vi "report.vi"() -> ()   [LabVIEW 2019, in "database.lvlib"]
uses:
  database.lvlib
  <vilib>/Utility/NIReport.llb/Report Type.ctl
  <vilib>/addons/_office/_exclsub.llb/font.ctl
  <vilib>/Utility/miscctls.llb/LVRowAndColumnTypeDef.ctl
  <vilib>/addons/_office/excel.llb/Excel Easy Table (str).vi
  <vilib>/Utility/NIReport.llb/NI_report.lvclass
  <vilib>/addons/_office/NI_ReportGenerationToolkit.lvlib
  <vilib>/Utility/NIReport.llb/NI_ReportGenerationCore.lvlib
panel:
  in  "Tab Control 1":T1(tab)
  in  "Tab Control 2":T2(tab)
  out "Grading Table Disc 1":string[][](table)
  out "Grading Table Disc 2":string[][](table)
  out "Grading Table Disc 3":string[][](table)
  out "Grading Table Disc 4":string[][](table)
  out "Grading Table Disc 5":string[][](table)
  out "Grading Table Disc 6":string[][](table)
  in  "Search 1":bool
  in  "Print 1":bool
  in  "Close 1":bool
  in  "Save 1":bool
  in  "Tab Control 3":T2(tab)
  out "Main Grading Table Disc 1":string[][](table)
  out "Main Grading Table Disc 2":string[][](table)
  out "Main Grading Table Disc 3":string[][](table)
  out "Main Grading Table Disc 4":string[][](table)
  out "Main Grading Table Disc 5":string[][](table)
  out "Main Grading Table Disc 6":string[][](table)
  in  "Close 2":bool
  in  "Print 2":bool
  in  "Search 2":bool
  in  "Save 2":bool
  out "Log Table":string[][](table)
  out "Log Catalog Table":string[][](table)
  in  "Search 3":bool
  in  "Print 3":bool
  in  "Close 3":bool
  in  "Save 3":bool
  out "User Table":string[][](table)
  in  "Close 4":bool
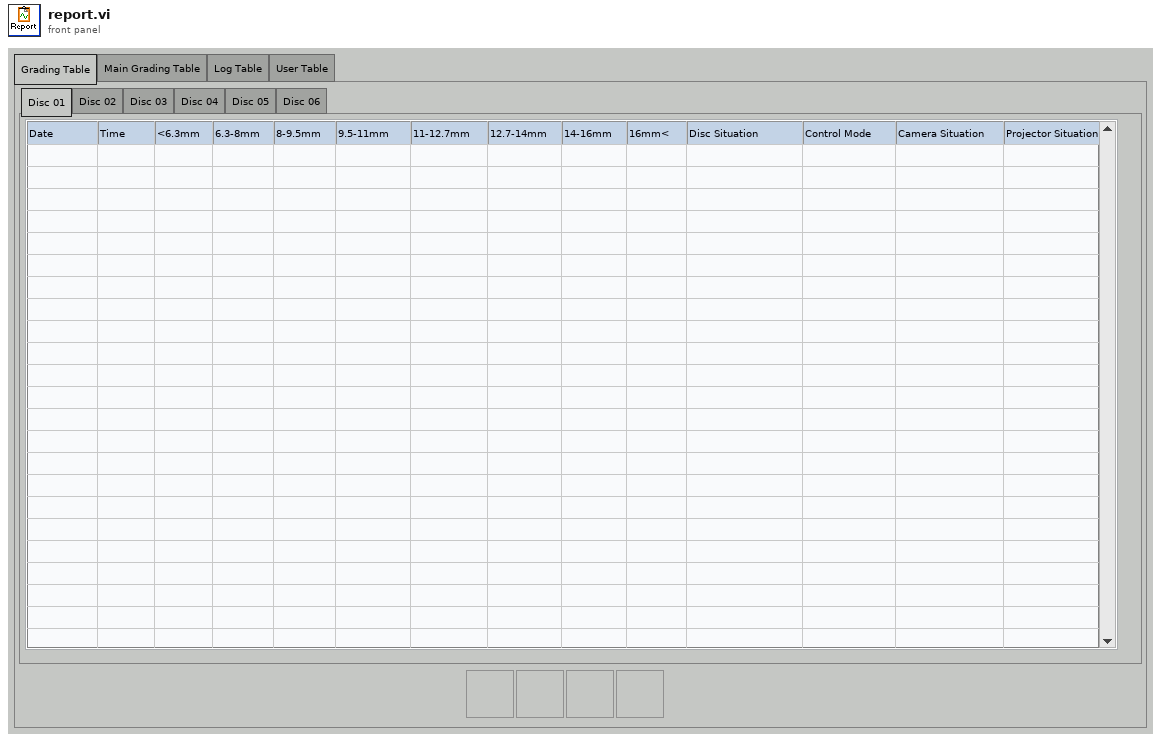
[diagram p1: front panel]
types:
  T1 = enum32{"Grading Table", "Main Grading Table", "Log Table", "User Table"}
  T2 = enum32{"Disc 01", "Disc 02", "Disc 03", "Disc 04", "Disc 05", "Disc 06"}
  T3 = enum16{"None", "On Hover", "On Key Focus", "On Hover or Key Focus"}
  T4 = typedef "NI_ReportGenerationToolkit.lvlib/font.ctl" = cluster{"font name":string, "font size":dbl, "bold":u16, "italic":u16, "underline":u16, "strike through":u16, "font color":u32}
  T5 = typedef "NI_ReportGenerationCore.lvlib/Report Type.ctl" = enum16{"HTML", "Word", "Excel"}
  T6 = enum16{"maximized", "minimized", "normal", "no change"}
  T7 = typedef "LVRowAndColumnTypeDef.ctl" = cluster{"Row":i32, "Column":i32}
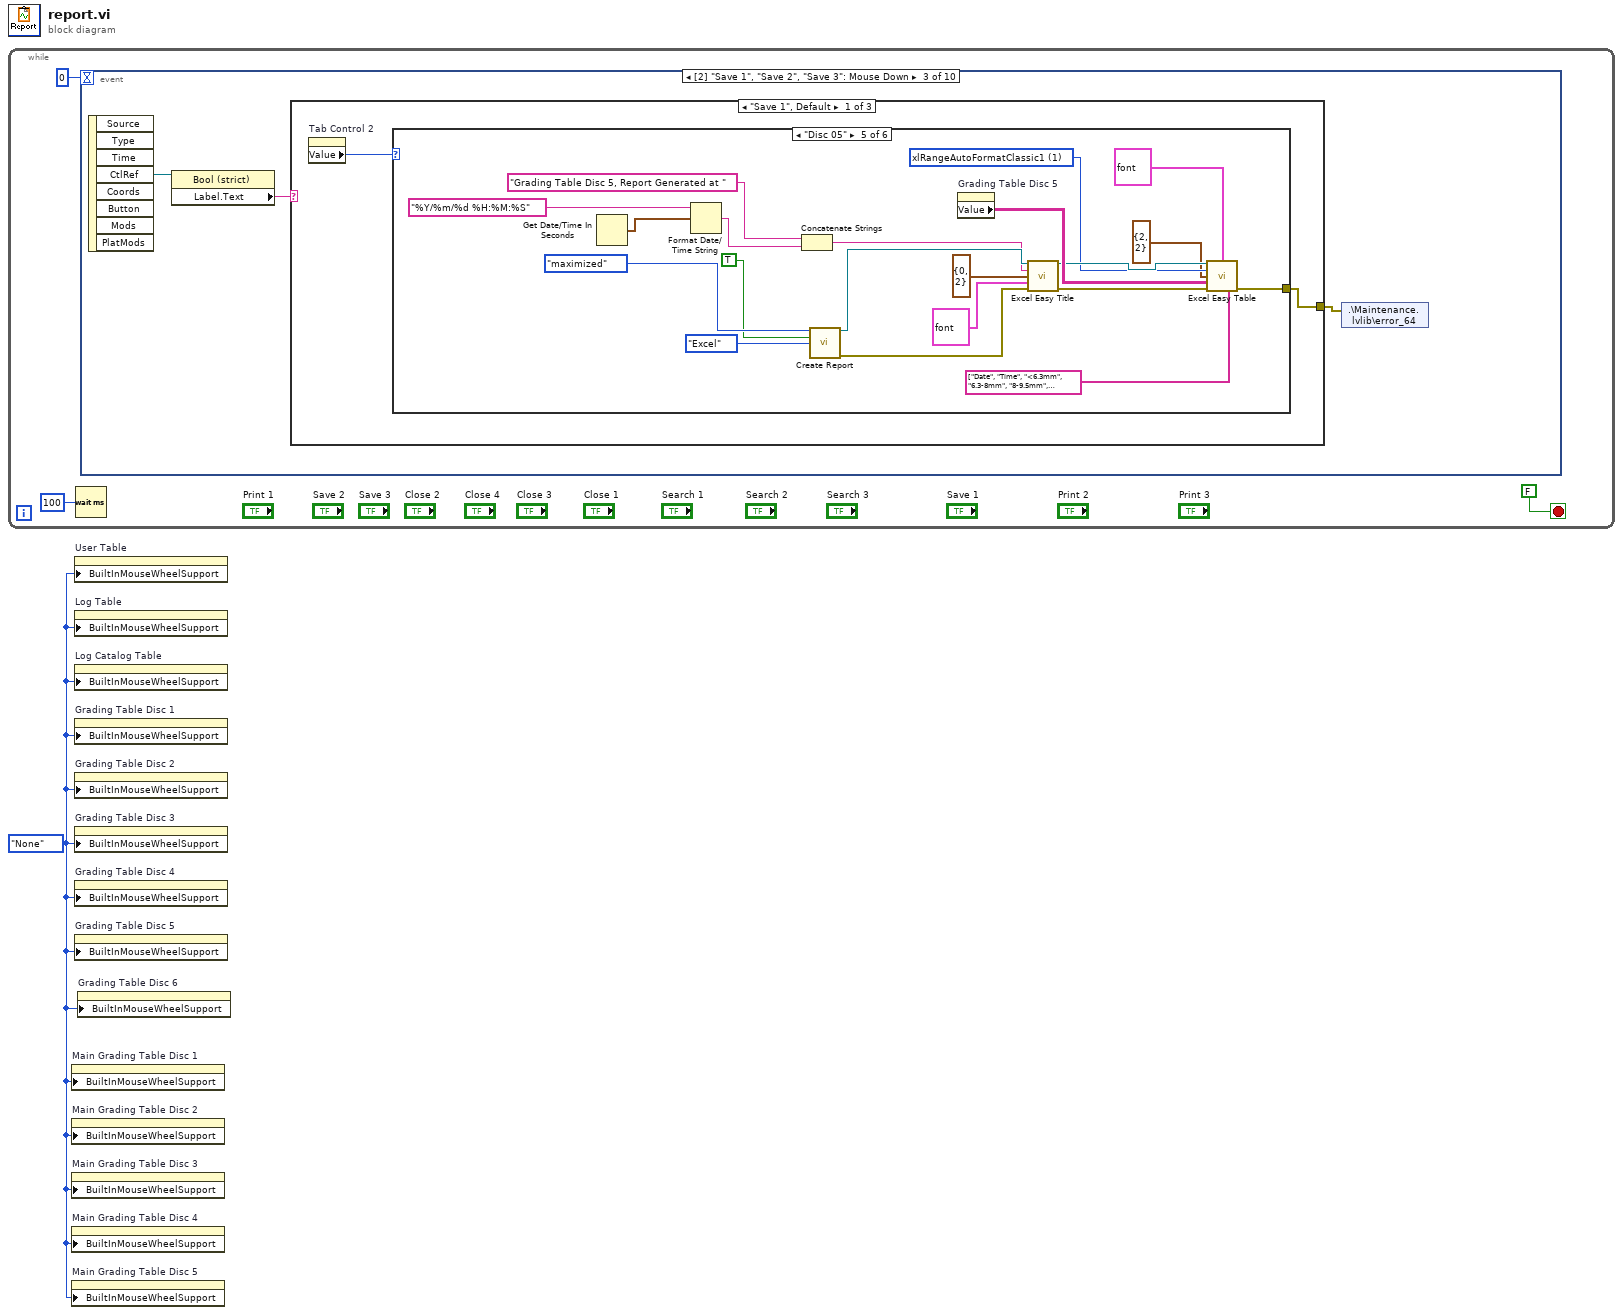
[diagram p0: block diagram]
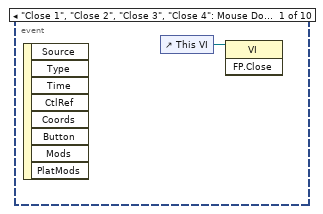
[diagram p2: hidden frame]
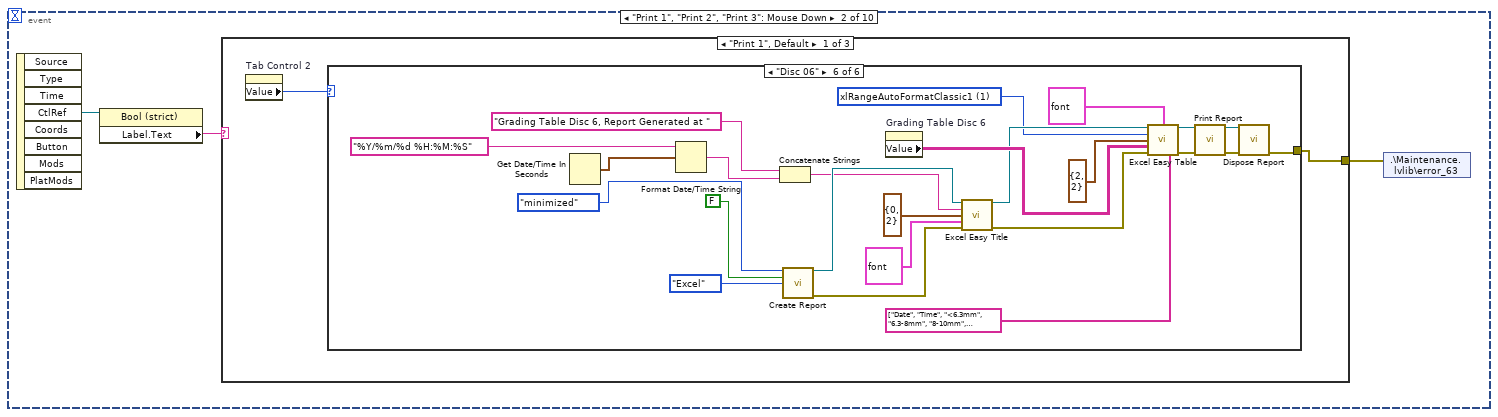
[diagram p3: hidden frame]
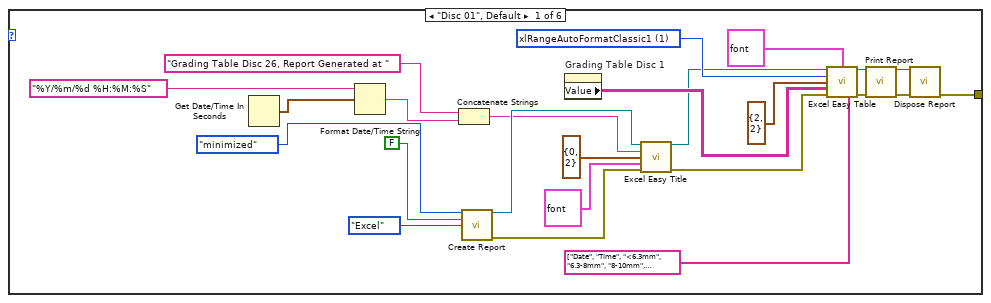
[diagram p4: hidden frame]
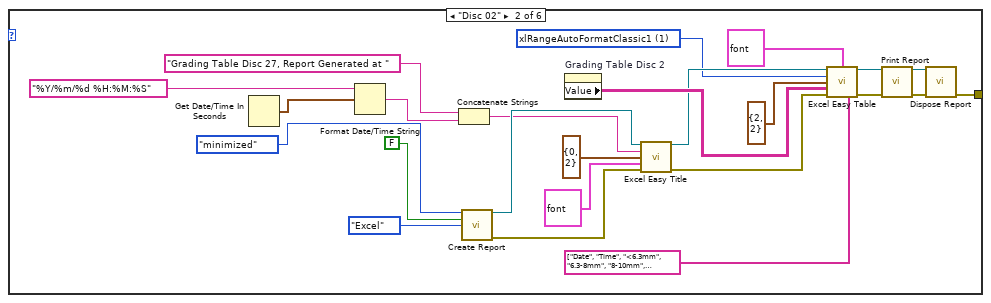
[diagram p5: hidden frame]
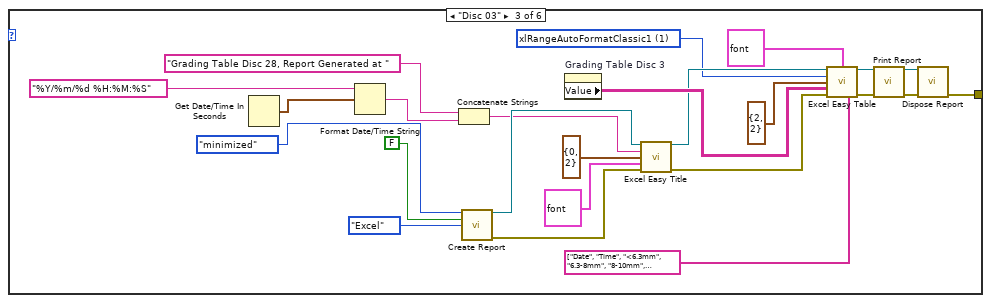
[diagram p6: hidden frame]
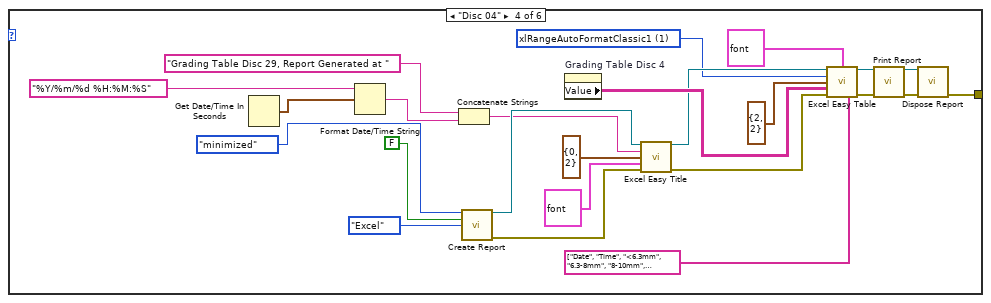
[diagram p7: hidden frame]
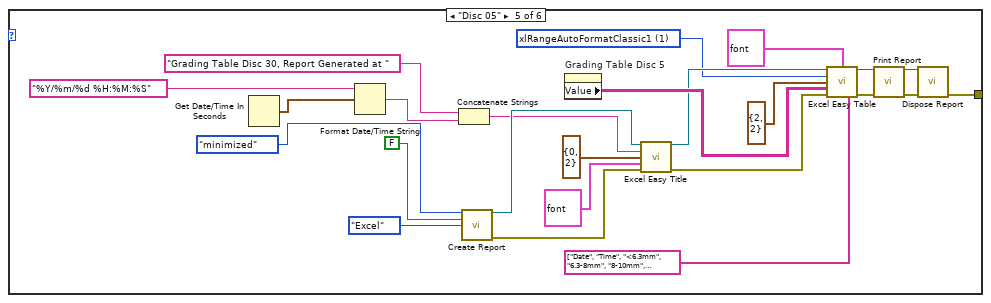
[diagram p8: hidden frame]
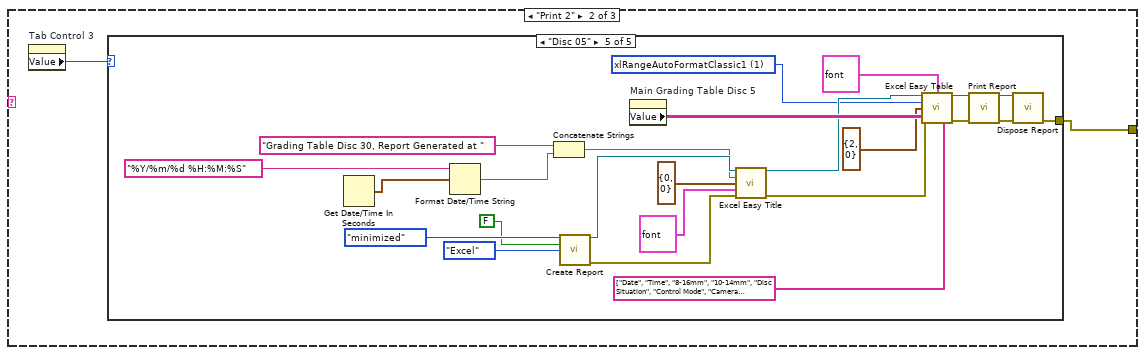
[diagram p9: hidden frame]
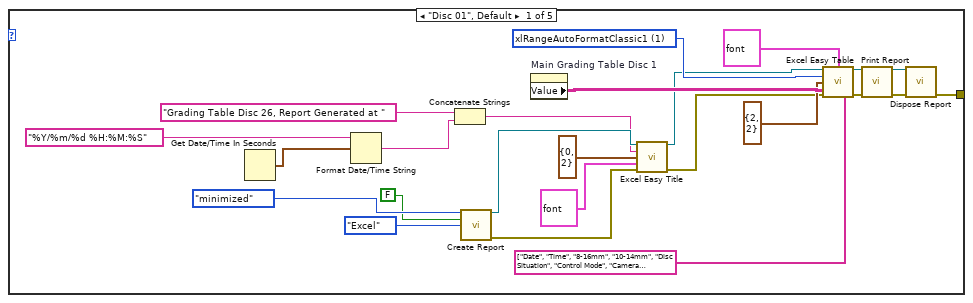
[diagram p10: hidden frame]
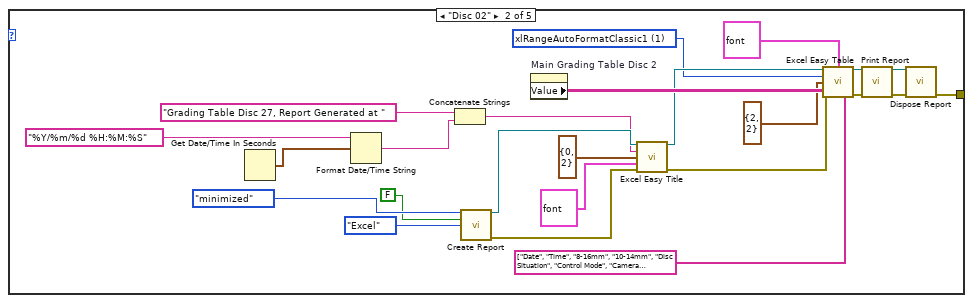
[diagram p11: hidden frame]
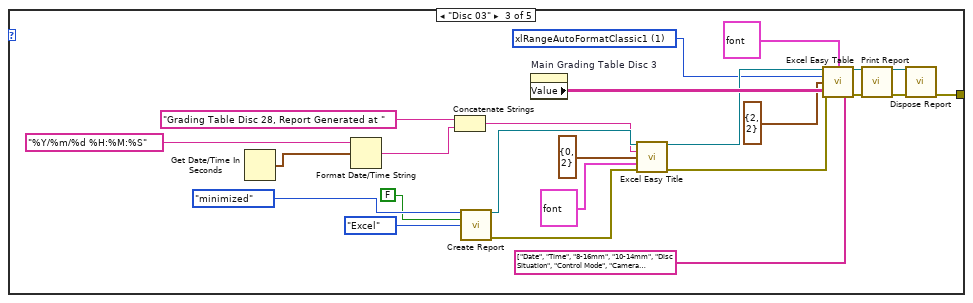
[diagram p12: hidden frame]
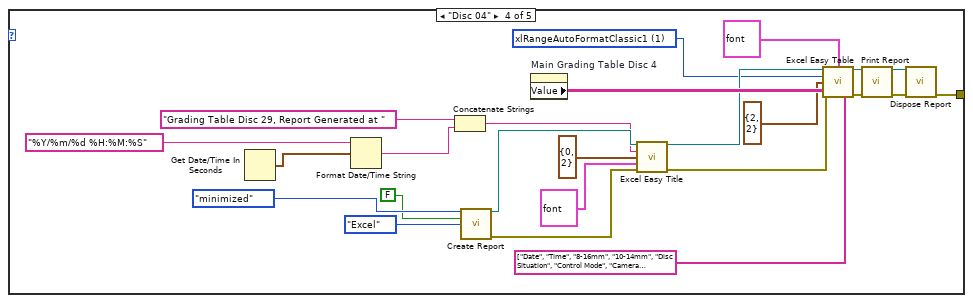
[diagram p13: hidden frame]
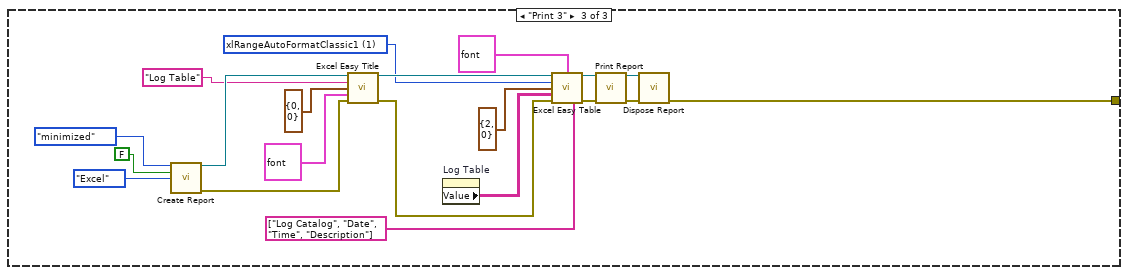
[diagram p14: hidden frame]
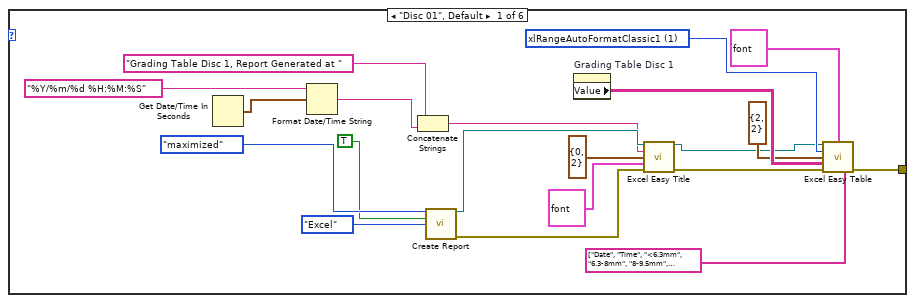
[diagram p15: hidden frame]
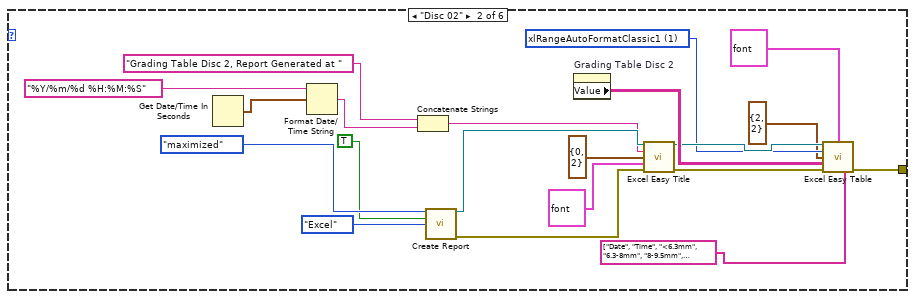
[diagram p16: hidden frame]
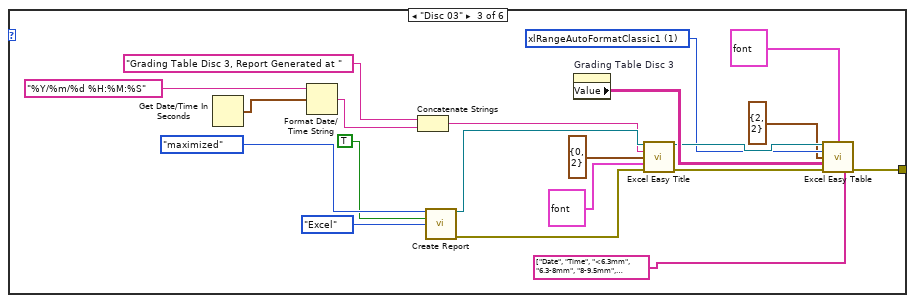
[diagram p17: hidden frame]
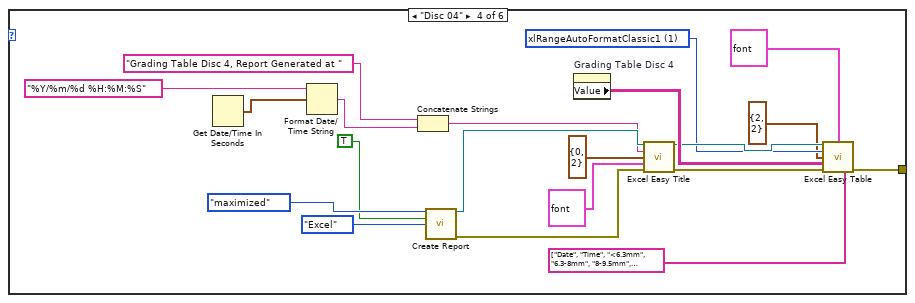
[diagram p18: hidden frame]
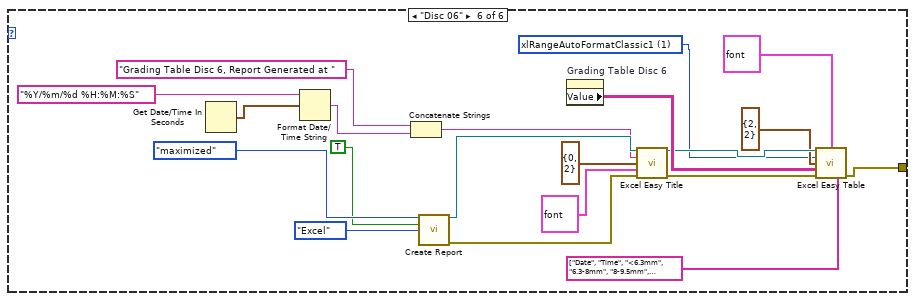
[diagram p19: hidden frame]
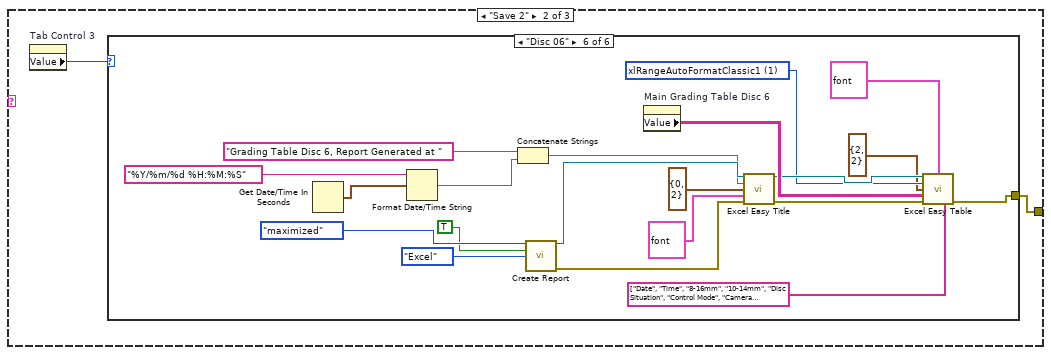
[diagram p20: hidden frame]
diagram:
  w1 = T3."None" ("Built-In Mouse Wheel Support")
  n1 = while {
    stop <- FALSE stop-if-true
    n2 = Wait (ms)(milliseconds to wait=u32 100) -> ()  [unwired: 1 out]
    n3 = event shown="[2] \"Save 1\", \"Save 2\", \"Save 3\": Mouse Down" {
      selector: _ -> [_ _ _ _ _ _ _ _ _ _]
      dyn-events: _ -> [_ _ _ _ _ _ _ _ _ _]
      timeout: 0 -> [_ _ _ _ _ _ _ _ _ _]
      event "Close 1", "Close 2", "Close 3", "Close 4": Mouse Down {
        n4 = event-data() -> ()  [unwired: 1 in, 8 out]
        n5 = control-ref of="This VI"() -> (w5:refnum<vi>)
        n6 = invoke class="VI" method="FP.Close"(reference=w5) -> ()  [unwired: 2 in, 3 out]
      }
      event "Print 1", "Print 2", "Print 3": Mouse Down {
        n7 = event-data() -> ("CtlRef"=w8:refnum<vi>)  [unwired: 1 in, 7 out]
        n8 = property class="Bool (strict)"(reference=w8) -> ("Label.Text"=w7:string)  [unwired: 1 in, 2 out]
        n9 = case shown="\"Print 1\", Default" w7 {
          tunnel: [w9 w155 w277] -> w6
          frame "Print 1", Default {
            n10 = property on="Tab Control 2" class="TabCtl (strict)"() -> ("Value"=w10:T2)  [unwired: 2 in, 2 out]
            n11 = case shown="\"Disc 06\"" w10 {
              tunnel: [w11 w35 w59 w83 w107 w131] -> w9
              frame "Disc 01", Default {
                w28 = 1 items=["xlRangeAutoFormat3DEffects1"=13, "xlRangeAutoFormat3DEffects2"=14, "xlRangeAutoFormatAccounting1"=4, "xlRangeAutoFormatAccounting2"=5, "xlRangeAutoFormatAccounting3"=6, "xlRangeAutoFormatAccounting4"=17, "xlRangeAutoFormatClassic1"=1, "xlRangeAutoFormatClassic2"=2, "xlRangeAutoFormatClassic3"=3, "xlRangeAutoFormatColor1"=7, "xlRangeAutoFormatColor2"=8, "xlRangeAutoFormatColor3"=9, "xlRangeAutoFormatList1"=10, "xlRangeAutoFormatList2"=11, "xlRangeAutoFormatList3"=12, "xlRangeAutoFormatLocalFormat1"=15, "xlRangeAutoFormatLocalFormat2"=16, "xlRangeAutoFormatLocalFormat3"=19, "xlRangeAutoFormatLocalFormat4"=20, "xlRangeAutoFormatReport1"=21, "xlRangeAutoFormatReport2"=22, "xlRangeAutoFormatReport3"=23, "xlRangeAutoFormatReport4"=24, "xlRangeAutoFormatReport5"=25, "xlRangeAutoFormatReport6"=26, "xlRangeAutoFormatReport7"=27, "xlRangeAutoFormatReport8"=28, "xlRangeAutoFormatReport9"=29, "xlRangeAutoFormatReport10"=30, "xlRangeAutoFormatClassicPivotTable"=31, "xlRangeAutoFormatTable1"=32, "xlRangeAutoFormatTable2"=33, "xlRangeAutoFormatTable3"=34, "xlRangeAutoFormatTable4"=35, "xlRangeAutoFormatTable5"=36, "xlRangeAutoFormatTable6"=37, "xlRangeAutoFormatTable7"=38, "xlRangeAutoFormatTable8"=39, "xlRangeAutoFormatTable9"=40, "xlRangeAutoFormatTable10"=41, "xlRangeAutoFormatPTNone"=42, "xlRangeAutoFormatNone"=-4142, "xlRangeAutoFormatSimple"=-4154] ("auto format (none)")
                n12 = Get Date/Time In Seconds() -> (seconds since 1Jan1904=w17:timestamp)
                n13 = Format Date/Time String(time format string (%c)="%Y/%m/%d %H:%M:%S", seconds (now)=w17) -> (date/time string=w18:string)  [unwired: 1 in]
                n14 = Concatenate Strings("Grading Table Disc 26, Report Generated at " ("title"), w18) -> (w19:string)
                n15 = call <vilib>:"Create Report.vi"("window state (normal)"=T6."minimized", "display alerts? (F)"=FALSE, "report type"=Report_Type."Excel") -> ("report out"=w24:refnum<class "NI_report.lvclass">, "error out"=w26:errorcluster)  [unwired: 11 in]
                n16 = property on="Grading Table Disc 1" class="Tbl (strict)"() -> ("Value"=w32:string[][])  [unwired: 2 in, 2 out]
                n17 = call <vilib>:"Excel Easy Title.vi"("report in"=w24, "title"=w19, "start (0, 0)"=cluster{"row":i32, "column":i32} {"row"=0, "column"=2}, "font"=T4 {"font name"="Times New Roman", "font size"=24.0, "bold"=1, "italic"=0, "underline"=0, "strike through"=0, "font color"=16777216}, "error in (no error)"=w26) -> ("report out"=w23:refnum<class "NI_report.lvclass">, "error out"=w25:errorcluster)  [unwired: 8 in, 1 out]
                n18 = call-poly <vilib>:"Excel Easy Table.vi"("report in"=w23, "font"=T4 {"font name"="Times New Roman", "font size"=12.0, "bold"=0, "italic"=0, "underline"=0, "strike through"=0, "font color"=16777216}, "auto format (none)"=w28, "start (0, 0)"=cluster{"row":i32, "column":i32} {"row"=2, "column"=2}, "text data"=w32, "error in (no error)"=w25, "column headers"=string[] ["Date", "Time", "<6.3mm", "6.3-8mm", "8-10mm", "10-12.5mm", "12.5-14mm", "14-16mm", "16-18mm", "18mm<", "Disc Situation", "Control Mode", "Camera Situation", "Projector Situation"]) -> ("report out"=w15:refnum<class "NI_report.lvclass">, "error out"=w14:errorcluster)  [unwired: 4 in, 3 out]
                n19 = call-dynamic "Print Report.vi"("report in"=w15, "error in (no error)"=w14) -> ("report out"=w13:refnum<class "NI_report.lvclass">, "error out"=w12:errorcluster)  [unwired: 12 in]
                n20 = call-dynamic "Dispose Report.vi"("report in"=w13, "error in (no error)"=w12) -> ("error out"=w11:errorcluster)  [unwired: 13 in]
              }
              frame "Disc 02" {
                w42 = 1 items=["xlRangeAutoFormat3DEffects1"=13, "xlRangeAutoFormat3DEffects2"=14, "xlRangeAutoFormatAccounting1"=4, "xlRangeAutoFormatAccounting2"=5, "xlRangeAutoFormatAccounting3"=6, "xlRangeAutoFormatAccounting4"=17, "xlRangeAutoFormatClassic1"=1, "xlRangeAutoFormatClassic2"=2, "xlRangeAutoFormatClassic3"=3, "xlRangeAutoFormatColor1"=7, "xlRangeAutoFormatColor2"=8, "xlRangeAutoFormatColor3"=9, "xlRangeAutoFormatList1"=10, "xlRangeAutoFormatList2"=11, "xlRangeAutoFormatList3"=12, "xlRangeAutoFormatLocalFormat1"=15, "xlRangeAutoFormatLocalFormat2"=16, "xlRangeAutoFormatLocalFormat3"=19, "xlRangeAutoFormatLocalFormat4"=20, "xlRangeAutoFormatReport1"=21, "xlRangeAutoFormatReport2"=22, "xlRangeAutoFormatReport3"=23, "xlRangeAutoFormatReport4"=24, "xlRangeAutoFormatReport5"=25, "xlRangeAutoFormatReport6"=26, "xlRangeAutoFormatReport7"=27, "xlRangeAutoFormatReport8"=28, "xlRangeAutoFormatReport9"=29, "xlRangeAutoFormatReport10"=30, "xlRangeAutoFormatClassicPivotTable"=31, "xlRangeAutoFormatTable1"=32, "xlRangeAutoFormatTable2"=33, "xlRangeAutoFormatTable3"=34, "xlRangeAutoFormatTable4"=35, "xlRangeAutoFormatTable5"=36, "xlRangeAutoFormatTable6"=37, "xlRangeAutoFormatTable7"=38, "xlRangeAutoFormatTable8"=39, "xlRangeAutoFormatTable9"=40, "xlRangeAutoFormatTable10"=41, "xlRangeAutoFormatPTNone"=42, "xlRangeAutoFormatNone"=-4142, "xlRangeAutoFormatSimple"=-4154] ("auto format (none)")
                n21 = Get Date/Time In Seconds() -> (seconds since 1Jan1904=w51:timestamp)
                n22 = Format Date/Time String(time format string (%c)="%Y/%m/%d %H:%M:%S", seconds (now)=w51) -> (date/time string=w52:string)  [unwired: 1 in]
                n23 = Concatenate Strings("Grading Table Disc 27, Report Generated at " ("title"), w52) -> (w53:string)
                n24 = call <vilib>:"Create Report.vi"("window state (normal)"=T6."minimized", "display alerts? (F)"=FALSE, "report type"=Report_Type."Excel") -> ("report out"=w55:refnum<class "NI_report.lvclass">, "error out"=w57:errorcluster)  [unwired: 11 in]
                n25 = property on="Grading Table Disc 2" class="Tbl (strict)"() -> ("Value"=w58:string[][])  [unwired: 2 in, 2 out]
                n26 = call <vilib>:"Excel Easy Title.vi"("report in"=w55, "title"=w53, "start (0, 0)"=cluster{"row":i32, "column":i32} {"row"=0, "column"=2}, "font"=T4 {"font name"="Times New Roman", "font size"=24.0, "bold"=1, "italic"=0, "underline"=0, "strike through"=0, "font color"=16777216}, "error in (no error)"=w57) -> ("report out"=w54:refnum<class "NI_report.lvclass">, "error out"=w56:errorcluster)  [unwired: 8 in, 1 out]
                n27 = call-poly <vilib>:"Excel Easy Table.vi"("report in"=w54, "font"=T4 {"font name"="Times New Roman", "font size"=12.0, "bold"=0, "italic"=0, "underline"=0, "strike through"=0, "font color"=16777216}, "auto format (none)"=w42, "start (0, 0)"=cluster{"row":i32, "column":i32} {"row"=2, "column"=2}, "text data"=w58, "error in (no error)"=w56, "column headers"=string[] ["Date", "Time", "<6.3mm", "6.3-8mm", "8-10mm", "10-12.5mm", "12.5-14mm", "14-16mm", "16-18mm", "18mm<", "Disc Situation", "Control Mode", "Camera Situation", "Projector Situation"]) -> ("report out"=w39:refnum<class "NI_report.lvclass">, "error out"=w38:errorcluster)  [unwired: 4 in, 3 out]
                n28 = call-dynamic "Print Report.vi"("report in"=w39, "error in (no error)"=w38) -> ("report out"=w36:refnum<class "NI_report.lvclass">, "error out"=w37:errorcluster)  [unwired: 12 in]
                n29 = call-dynamic "Dispose Report.vi"("report in"=w36, "error in (no error)"=w37) -> ("error out"=w35:errorcluster)  [unwired: 13 in]
              }
              frame "Disc 03" {
                w66 = 1 items=["xlRangeAutoFormat3DEffects1"=13, "xlRangeAutoFormat3DEffects2"=14, "xlRangeAutoFormatAccounting1"=4, "xlRangeAutoFormatAccounting2"=5, "xlRangeAutoFormatAccounting3"=6, "xlRangeAutoFormatAccounting4"=17, "xlRangeAutoFormatClassic1"=1, "xlRangeAutoFormatClassic2"=2, "xlRangeAutoFormatClassic3"=3, "xlRangeAutoFormatColor1"=7, "xlRangeAutoFormatColor2"=8, "xlRangeAutoFormatColor3"=9, "xlRangeAutoFormatList1"=10, "xlRangeAutoFormatList2"=11, "xlRangeAutoFormatList3"=12, "xlRangeAutoFormatLocalFormat1"=15, "xlRangeAutoFormatLocalFormat2"=16, "xlRangeAutoFormatLocalFormat3"=19, "xlRangeAutoFormatLocalFormat4"=20, "xlRangeAutoFormatReport1"=21, "xlRangeAutoFormatReport2"=22, "xlRangeAutoFormatReport3"=23, "xlRangeAutoFormatReport4"=24, "xlRangeAutoFormatReport5"=25, "xlRangeAutoFormatReport6"=26, "xlRangeAutoFormatReport7"=27, "xlRangeAutoFormatReport8"=28, "xlRangeAutoFormatReport9"=29, "xlRangeAutoFormatReport10"=30, "xlRangeAutoFormatClassicPivotTable"=31, "xlRangeAutoFormatTable1"=32, "xlRangeAutoFormatTable2"=33, "xlRangeAutoFormatTable3"=34, "xlRangeAutoFormatTable4"=35, "xlRangeAutoFormatTable5"=36, "xlRangeAutoFormatTable6"=37, "xlRangeAutoFormatTable7"=38, "xlRangeAutoFormatTable8"=39, "xlRangeAutoFormatTable9"=40, "xlRangeAutoFormatTable10"=41, "xlRangeAutoFormatPTNone"=42, "xlRangeAutoFormatNone"=-4142, "xlRangeAutoFormatSimple"=-4154] ("auto format (none)")
                n30 = Get Date/Time In Seconds() -> (seconds since 1Jan1904=w75:timestamp)
                n31 = Format Date/Time String(time format string (%c)="%Y/%m/%d %H:%M:%S", seconds (now)=w75) -> (date/time string=w76:string)  [unwired: 1 in]
                n32 = Concatenate Strings("Grading Table Disc 28, Report Generated at " ("title"), w76) -> (w77:string)
                n33 = call <vilib>:"Create Report.vi"("window state (normal)"=T6."minimized", "display alerts? (F)"=FALSE, "report type"=Report_Type."Excel") -> ("report out"=w79:refnum<class "NI_report.lvclass">, "error out"=w81:errorcluster)  [unwired: 11 in]
                n34 = property on="Grading Table Disc 3" class="Tbl (strict)"() -> ("Value"=w82:string[][])  [unwired: 2 in, 2 out]
                n35 = call <vilib>:"Excel Easy Title.vi"("report in"=w79, "title"=w77, "start (0, 0)"=cluster{"row":i32, "column":i32} {"row"=0, "column"=2}, "font"=T4 {"font name"="Times New Roman", "font size"=24.0, "bold"=1, "italic"=0, "underline"=0, "strike through"=0, "font color"=16777216}, "error in (no error)"=w81) -> ("report out"=w78:refnum<class "NI_report.lvclass">, "error out"=w80:errorcluster)  [unwired: 8 in, 1 out]
                n36 = call-poly <vilib>:"Excel Easy Table.vi"("report in"=w78, "font"=T4 {"font name"="Times New Roman", "font size"=12.0, "bold"=0, "italic"=0, "underline"=0, "strike through"=0, "font color"=16777216}, "auto format (none)"=w66, "start (0, 0)"=cluster{"row":i32, "column":i32} {"row"=2, "column"=2}, "text data"=w82, "error in (no error)"=w80, "column headers"=string[] ["Date", "Time", "<6.3mm", "6.3-8mm", "8-10mm", "10-12.5mm", "12.5-14mm", "14-16mm", "16-18mm", "18mm<", "Disc Situation", "Control Mode", "Camera Situation", "Projector Situation"]) -> ("report out"=w63:refnum<class "NI_report.lvclass">, "error out"=w62:errorcluster)  [unwired: 4 in, 3 out]
                n37 = call-dynamic "Print Report.vi"("report in"=w63, "error in (no error)"=w62) -> ("report out"=w60:refnum<class "NI_report.lvclass">, "error out"=w61:errorcluster)  [unwired: 12 in]
                n38 = call-dynamic "Dispose Report.vi"("report in"=w60, "error in (no error)"=w61) -> ("error out"=w59:errorcluster)  [unwired: 13 in]
              }
              frame "Disc 04" {
                w90 = 1 items=["xlRangeAutoFormat3DEffects1"=13, "xlRangeAutoFormat3DEffects2"=14, "xlRangeAutoFormatAccounting1"=4, "xlRangeAutoFormatAccounting2"=5, "xlRangeAutoFormatAccounting3"=6, "xlRangeAutoFormatAccounting4"=17, "xlRangeAutoFormatClassic1"=1, "xlRangeAutoFormatClassic2"=2, "xlRangeAutoFormatClassic3"=3, "xlRangeAutoFormatColor1"=7, "xlRangeAutoFormatColor2"=8, "xlRangeAutoFormatColor3"=9, "xlRangeAutoFormatList1"=10, "xlRangeAutoFormatList2"=11, "xlRangeAutoFormatList3"=12, "xlRangeAutoFormatLocalFormat1"=15, "xlRangeAutoFormatLocalFormat2"=16, "xlRangeAutoFormatLocalFormat3"=19, "xlRangeAutoFormatLocalFormat4"=20, "xlRangeAutoFormatReport1"=21, "xlRangeAutoFormatReport2"=22, "xlRangeAutoFormatReport3"=23, "xlRangeAutoFormatReport4"=24, "xlRangeAutoFormatReport5"=25, "xlRangeAutoFormatReport6"=26, "xlRangeAutoFormatReport7"=27, "xlRangeAutoFormatReport8"=28, "xlRangeAutoFormatReport9"=29, "xlRangeAutoFormatReport10"=30, "xlRangeAutoFormatClassicPivotTable"=31, "xlRangeAutoFormatTable1"=32, "xlRangeAutoFormatTable2"=33, "xlRangeAutoFormatTable3"=34, "xlRangeAutoFormatTable4"=35, "xlRangeAutoFormatTable5"=36, "xlRangeAutoFormatTable6"=37, "xlRangeAutoFormatTable7"=38, "xlRangeAutoFormatTable8"=39, "xlRangeAutoFormatTable9"=40, "xlRangeAutoFormatTable10"=41, "xlRangeAutoFormatPTNone"=42, "xlRangeAutoFormatNone"=-4142, "xlRangeAutoFormatSimple"=-4154] ("auto format (none)")
                n39 = Get Date/Time In Seconds() -> (seconds since 1Jan1904=w99:timestamp)
                n40 = Format Date/Time String(time format string (%c)="%Y/%m/%d %H:%M:%S", seconds (now)=w99) -> (date/time string=w100:string)  [unwired: 1 in]
                n41 = Concatenate Strings("Grading Table Disc 29, Report Generated at " ("title"), w100) -> (w101:string)
                n42 = call <vilib>:"Create Report.vi"("window state (normal)"=T6."minimized", "display alerts? (F)"=FALSE, "report type"=Report_Type."Excel") -> ("report out"=w103:refnum<class "NI_report.lvclass">, "error out"=w105:errorcluster)  [unwired: 11 in]
                n43 = property on="Grading Table Disc 4" class="Tbl (strict)"() -> ("Value"=w106:string[][])  [unwired: 2 in, 2 out]
                n44 = call <vilib>:"Excel Easy Title.vi"("report in"=w103, "title"=w101, "start (0, 0)"=cluster{"row":i32, "column":i32} {"row"=0, "column"=2}, "font"=T4 {"font name"="Times New Roman", "font size"=24.0, "bold"=1, "italic"=0, "underline"=0, "strike through"=0, "font color"=16777216}, "error in (no error)"=w105) -> ("report out"=w102:refnum<class "NI_report.lvclass">, "error out"=w104:errorcluster)  [unwired: 8 in, 1 out]
                n45 = call-poly <vilib>:"Excel Easy Table.vi"("report in"=w102, "font"=T4 {"font name"="Times New Roman", "font size"=12.0, "bold"=0, "italic"=0, "underline"=0, "strike through"=0, "font color"=16777216}, "auto format (none)"=w90, "start (0, 0)"=cluster{"row":i32, "column":i32} {"row"=2, "column"=2}, "text data"=w106, "error in (no error)"=w104, "column headers"=string[] ["Date", "Time", "<6.3mm", "6.3-8mm", "8-10mm", "10-12.5mm", "12.5-14mm", "14-16mm", "16-18mm", "18mm<", "Disc Situation", "Control Mode", "Camera Situation", "Projector Situation"]) -> ("report out"=w87:refnum<class "NI_report.lvclass">, "error out"=w86:errorcluster)  [unwired: 4 in, 3 out]
                n46 = call-dynamic "Print Report.vi"("report in"=w87, "error in (no error)"=w86) -> ("report out"=w84:refnum<class "NI_report.lvclass">, "error out"=w85:errorcluster)  [unwired: 12 in]
                n47 = call-dynamic "Dispose Report.vi"("report in"=w84, "error in (no error)"=w85) -> ("error out"=w83:errorcluster)  [unwired: 13 in]
              }
              frame "Disc 05" {
                w114 = 1 items=["xlRangeAutoFormat3DEffects1"=13, "xlRangeAutoFormat3DEffects2"=14, "xlRangeAutoFormatAccounting1"=4, "xlRangeAutoFormatAccounting2"=5, "xlRangeAutoFormatAccounting3"=6, "xlRangeAutoFormatAccounting4"=17, "xlRangeAutoFormatClassic1"=1, "xlRangeAutoFormatClassic2"=2, "xlRangeAutoFormatClassic3"=3, "xlRangeAutoFormatColor1"=7, "xlRangeAutoFormatColor2"=8, "xlRangeAutoFormatColor3"=9, "xlRangeAutoFormatList1"=10, "xlRangeAutoFormatList2"=11, "xlRangeAutoFormatList3"=12, "xlRangeAutoFormatLocalFormat1"=15, "xlRangeAutoFormatLocalFormat2"=16, "xlRangeAutoFormatLocalFormat3"=19, "xlRangeAutoFormatLocalFormat4"=20, "xlRangeAutoFormatReport1"=21, "xlRangeAutoFormatReport2"=22, "xlRangeAutoFormatReport3"=23, "xlRangeAutoFormatReport4"=24, "xlRangeAutoFormatReport5"=25, "xlRangeAutoFormatReport6"=26, "xlRangeAutoFormatReport7"=27, "xlRangeAutoFormatReport8"=28, "xlRangeAutoFormatReport9"=29, "xlRangeAutoFormatReport10"=30, "xlRangeAutoFormatClassicPivotTable"=31, "xlRangeAutoFormatTable1"=32, "xlRangeAutoFormatTable2"=33, "xlRangeAutoFormatTable3"=34, "xlRangeAutoFormatTable4"=35, "xlRangeAutoFormatTable5"=36, "xlRangeAutoFormatTable6"=37, "xlRangeAutoFormatTable7"=38, "xlRangeAutoFormatTable8"=39, "xlRangeAutoFormatTable9"=40, "xlRangeAutoFormatTable10"=41, "xlRangeAutoFormatPTNone"=42, "xlRangeAutoFormatNone"=-4142, "xlRangeAutoFormatSimple"=-4154] ("auto format (none)")
                n48 = Get Date/Time In Seconds() -> (seconds since 1Jan1904=w123:timestamp)
                n49 = Format Date/Time String(time format string (%c)="%Y/%m/%d %H:%M:%S", seconds (now)=w123) -> (date/time string=w124:string)  [unwired: 1 in]
                n50 = Concatenate Strings("Grading Table Disc 30, Report Generated at " ("title"), w124) -> (w125:string)
                n51 = call <vilib>:"Create Report.vi"("window state (normal)"=T6."minimized", "display alerts? (F)"=FALSE, "report type"=Report_Type."Excel") -> ("report out"=w127:refnum<class "NI_report.lvclass">, "error out"=w129:errorcluster)  [unwired: 11 in]
                n52 = property on="Grading Table Disc 5" class="Tbl (strict)"() -> ("Value"=w130:string[][])  [unwired: 2 in, 2 out]
                n53 = call <vilib>:"Excel Easy Title.vi"("report in"=w127, "title"=w125, "start (0, 0)"=cluster{"row":i32, "column":i32} {"row"=0, "column"=2}, "font"=T4 {"font name"="Times New Roman", "font size"=24.0, "bold"=1, "italic"=0, "underline"=0, "strike through"=0, "font color"=16777216}, "error in (no error)"=w129) -> ("report out"=w126:refnum<class "NI_report.lvclass">, "error out"=w128:errorcluster)  [unwired: 8 in, 1 out]
                n54 = call-poly <vilib>:"Excel Easy Table.vi"("report in"=w126, "font"=T4 {"font name"="Times New Roman", "font size"=12.0, "bold"=0, "italic"=0, "underline"=0, "strike through"=0, "font color"=16777216}, "auto format (none)"=w114, "start (0, 0)"=cluster{"row":i32, "column":i32} {"row"=2, "column"=2}, "text data"=w130, "error in (no error)"=w128, "column headers"=string[] ["Date", "Time", "<6.3mm", "6.3-8mm", "8-10mm", "10-12.5mm", "12.5-14mm", "14-16mm", "16-18mm", "18mm<", "Disc Situation", "Control Mode", "Camera Situation", "Projector Situation"]) -> ("report out"=w110:refnum<class "NI_report.lvclass">, "error out"=w111:errorcluster)  [unwired: 4 in, 3 out]
                n55 = call-dynamic "Print Report.vi"("report in"=w110, "error in (no error)"=w111) -> ("report out"=w108:refnum<class "NI_report.lvclass">, "error out"=w109:errorcluster)  [unwired: 12 in]
                n56 = call-dynamic "Dispose Report.vi"("report in"=w108, "error in (no error)"=w109) -> ("error out"=w107:errorcluster)  [unwired: 13 in]
              }
              frame "Disc 06" {
                w138 = 1 items=["xlRangeAutoFormat3DEffects1"=13, "xlRangeAutoFormat3DEffects2"=14, "xlRangeAutoFormatAccounting1"=4, "xlRangeAutoFormatAccounting2"=5, "xlRangeAutoFormatAccounting3"=6, "xlRangeAutoFormatAccounting4"=17, "xlRangeAutoFormatClassic1"=1, "xlRangeAutoFormatClassic2"=2, "xlRangeAutoFormatClassic3"=3, "xlRangeAutoFormatColor1"=7, "xlRangeAutoFormatColor2"=8, "xlRangeAutoFormatColor3"=9, "xlRangeAutoFormatList1"=10, "xlRangeAutoFormatList2"=11, "xlRangeAutoFormatList3"=12, "xlRangeAutoFormatLocalFormat1"=15, "xlRangeAutoFormatLocalFormat2"=16, "xlRangeAutoFormatLocalFormat3"=19, "xlRangeAutoFormatLocalFormat4"=20, "xlRangeAutoFormatReport1"=21, "xlRangeAutoFormatReport2"=22, "xlRangeAutoFormatReport3"=23, "xlRangeAutoFormatReport4"=24, "xlRangeAutoFormatReport5"=25, "xlRangeAutoFormatReport6"=26, "xlRangeAutoFormatReport7"=27, "xlRangeAutoFormatReport8"=28, "xlRangeAutoFormatReport9"=29, "xlRangeAutoFormatReport10"=30, "xlRangeAutoFormatClassicPivotTable"=31, "xlRangeAutoFormatTable1"=32, "xlRangeAutoFormatTable2"=33, "xlRangeAutoFormatTable3"=34, "xlRangeAutoFormatTable4"=35, "xlRangeAutoFormatTable5"=36, "xlRangeAutoFormatTable6"=37, "xlRangeAutoFormatTable7"=38, "xlRangeAutoFormatTable8"=39, "xlRangeAutoFormatTable9"=40, "xlRangeAutoFormatTable10"=41, "xlRangeAutoFormatPTNone"=42, "xlRangeAutoFormatNone"=-4142, "xlRangeAutoFormatSimple"=-4154] ("auto format (none)")
                n57 = Get Date/Time In Seconds() -> (seconds since 1Jan1904=w147:timestamp)
                n58 = Format Date/Time String(time format string (%c)="%Y/%m/%d %H:%M:%S", seconds (now)=w147) -> (date/time string=w148:string)  [unwired: 1 in]
                n59 = Concatenate Strings("Grading Table Disc 6, Report Generated at " ("title"), w148) -> (w149:string)
                n60 = call <vilib>:"Create Report.vi"("window state (normal)"=T6."minimized", "display alerts? (F)"=FALSE, "report type"=Report_Type."Excel") -> ("report out"=w151:refnum<class "NI_report.lvclass">, "error out"=w153:errorcluster)  [unwired: 11 in]
                n61 = property on="Grading Table Disc 6" class="Tbl (strict)"() -> ("Value"=w154:string[][])  [unwired: 2 in, 2 out]
                n62 = call <vilib>:"Excel Easy Title.vi"("report in"=w151, "title"=w149, "start (0, 0)"=cluster{"row":i32, "column":i32} {"row"=0, "column"=2}, "font"=T4 {"font name"="Times New Roman", "font size"=24.0, "bold"=1, "italic"=0, "underline"=0, "strike through"=0, "font color"=16777216}, "error in (no error)"=w153) -> ("report out"=w150:refnum<class "NI_report.lvclass">, "error out"=w152:errorcluster)  [unwired: 8 in, 1 out]
                n63 = call-poly <vilib>:"Excel Easy Table.vi"("report in"=w150, "font"=T4 {"font name"="Times New Roman", "font size"=12.0, "bold"=0, "italic"=0, "underline"=0, "strike through"=0, "font color"=16777216}, "auto format (none)"=w138, "start (0, 0)"=cluster{"row":i32, "column":i32} {"row"=2, "column"=2}, "text data"=w154, "error in (no error)"=w152, "column headers"=string[] ["Date", "Time", "<6.3mm", "6.3-8mm", "8-10mm", "10-12.5mm", "12.5-14mm", "14-16mm", "16-18mm", "18mm<", "Disc Situation", "Control Mode", "Camera Situation", "Projector Situation"]) -> ("report out"=w134:refnum<class "NI_report.lvclass">, "error out"=w135:errorcluster)  [unwired: 4 in, 3 out]
                n64 = call-dynamic "Print Report.vi"("report in"=w134, "error in (no error)"=w135) -> ("report out"=w132:refnum<class "NI_report.lvclass">, "error out"=w133:errorcluster)  [unwired: 12 in]
                n65 = call-dynamic "Dispose Report.vi"("report in"=w132, "error in (no error)"=w133) -> ("error out"=w131:errorcluster)  [unwired: 13 in]
              }
            }
          }
          frame "Print 2" {
            n66 = property on="Tab Control 3" class="TabCtl (strict)"() -> ("Value"=w156:T2)  [unwired: 2 in, 2 out]
            n67 = case shown="\"Disc 05\"" w156 {
              tunnel: [w157 w181 w205 w229 w253] -> w155
              frame "Disc 01", Default {
                w175 = 1 items=["xlRangeAutoFormat3DEffects1"=13, "xlRangeAutoFormat3DEffects2"=14, "xlRangeAutoFormatAccounting1"=4, "xlRangeAutoFormatAccounting2"=5, "xlRangeAutoFormatAccounting3"=6, "xlRangeAutoFormatAccounting4"=17, "xlRangeAutoFormatClassic1"=1, "xlRangeAutoFormatClassic2"=2, "xlRangeAutoFormatClassic3"=3, "xlRangeAutoFormatColor1"=7, "xlRangeAutoFormatColor2"=8, "xlRangeAutoFormatColor3"=9, "xlRangeAutoFormatList1"=10, "xlRangeAutoFormatList2"=11, "xlRangeAutoFormatList3"=12, "xlRangeAutoFormatLocalFormat1"=15, "xlRangeAutoFormatLocalFormat2"=16, "xlRangeAutoFormatLocalFormat3"=19, "xlRangeAutoFormatLocalFormat4"=20, "xlRangeAutoFormatReport1"=21, "xlRangeAutoFormatReport2"=22, "xlRangeAutoFormatReport3"=23, "xlRangeAutoFormatReport4"=24, "xlRangeAutoFormatReport5"=25, "xlRangeAutoFormatReport6"=26, "xlRangeAutoFormatReport7"=27, "xlRangeAutoFormatReport8"=28, "xlRangeAutoFormatReport9"=29, "xlRangeAutoFormatReport10"=30, "xlRangeAutoFormatClassicPivotTable"=31, "xlRangeAutoFormatTable1"=32, "xlRangeAutoFormatTable2"=33, "xlRangeAutoFormatTable3"=34, "xlRangeAutoFormatTable4"=35, "xlRangeAutoFormatTable5"=36, "xlRangeAutoFormatTable6"=37, "xlRangeAutoFormatTable7"=38, "xlRangeAutoFormatTable8"=39, "xlRangeAutoFormatTable9"=40, "xlRangeAutoFormatTable10"=41, "xlRangeAutoFormatPTNone"=42, "xlRangeAutoFormatNone"=-4142, "xlRangeAutoFormatSimple"=-4154] ("auto format (none)")
                n68 = Get Date/Time In Seconds() -> (seconds since 1Jan1904=w164:timestamp)
                n69 = Format Date/Time String(time format string (%c)="%Y/%m/%d %H:%M:%S", seconds (now)=w164) -> (date/time string=w165:string)  [unwired: 1 in]
                n70 = Concatenate Strings("Grading Table Disc 26, Report Generated at " ("title"), w165) -> (w166:string)
                n71 = call <vilib>:"Create Report.vi"("window state (normal)"=T6."minimized", "display alerts? (F)"=FALSE, "report type"=Report_Type."Excel") -> ("report out"=w171:refnum<class "NI_report.lvclass">, "error out"=w173:errorcluster)  [unwired: 11 in]
                n72 = property on="Main Grading Table Disc 1" class="Tbl (strict)"() -> ("Value"=w178:string[][])  [unwired: 2 in, 2 out]
                n73 = call <vilib>:"Excel Easy Title.vi"("report in"=w171, "title"=w166, "start (0, 0)"=cluster{"row":i32, "column":i32} {"row"=0, "column"=2}, "font"=T4 {"font name"="Times New Roman", "font size"=24.0, "bold"=1, "italic"=0, "underline"=0, "strike through"=0, "font color"=16777216}, "error in (no error)"=w173) -> ("report out"=w170:refnum<class "NI_report.lvclass">, "error out"=w172:errorcluster)  [unwired: 8 in, 1 out]
                n74 = call-poly <vilib>:"Excel Easy Table.vi"("report in"=w170, "font"=T4 {"font name"="Times New Roman", "font size"=12.0, "bold"=0, "italic"=0, "underline"=0, "strike through"=0, "font color"=16777216}, "auto format (none)"=w175, "start (0, 0)"=cluster{"row":i32, "column":i32} {"row"=2, "column"=2}, "text data"=w178, "error in (no error)"=w172, "column headers"=string[] ["Date", "Time", "8-16mm", "10-14mm", "Disc Situation", "Control Mode", "Camera Situation", "Projector Situation"]) -> ("report out"=w160:refnum<class "NI_report.lvclass">, "error out"=w161:errorcluster)  [unwired: 4 in, 3 out]
                n75 = call-dynamic "Print Report.vi"("report in"=w160, "error in (no error)"=w161) -> ("report out"=w158:refnum<class "NI_report.lvclass">, "error out"=w159:errorcluster)  [unwired: 12 in]
                n76 = call-dynamic "Dispose Report.vi"("report in"=w158, "error in (no error)"=w159) -> ("error out"=w157:errorcluster)  [unwired: 13 in]
              }
              frame "Disc 02" {
                w188 = 1 items=["xlRangeAutoFormat3DEffects1"=13, "xlRangeAutoFormat3DEffects2"=14, "xlRangeAutoFormatAccounting1"=4, "xlRangeAutoFormatAccounting2"=5, "xlRangeAutoFormatAccounting3"=6, "xlRangeAutoFormatAccounting4"=17, "xlRangeAutoFormatClassic1"=1, "xlRangeAutoFormatClassic2"=2, "xlRangeAutoFormatClassic3"=3, "xlRangeAutoFormatColor1"=7, "xlRangeAutoFormatColor2"=8, "xlRangeAutoFormatColor3"=9, "xlRangeAutoFormatList1"=10, "xlRangeAutoFormatList2"=11, "xlRangeAutoFormatList3"=12, "xlRangeAutoFormatLocalFormat1"=15, "xlRangeAutoFormatLocalFormat2"=16, "xlRangeAutoFormatLocalFormat3"=19, "xlRangeAutoFormatLocalFormat4"=20, "xlRangeAutoFormatReport1"=21, "xlRangeAutoFormatReport2"=22, "xlRangeAutoFormatReport3"=23, "xlRangeAutoFormatReport4"=24, "xlRangeAutoFormatReport5"=25, "xlRangeAutoFormatReport6"=26, "xlRangeAutoFormatReport7"=27, "xlRangeAutoFormatReport8"=28, "xlRangeAutoFormatReport9"=29, "xlRangeAutoFormatReport10"=30, "xlRangeAutoFormatClassicPivotTable"=31, "xlRangeAutoFormatTable1"=32, "xlRangeAutoFormatTable2"=33, "xlRangeAutoFormatTable3"=34, "xlRangeAutoFormatTable4"=35, "xlRangeAutoFormatTable5"=36, "xlRangeAutoFormatTable6"=37, "xlRangeAutoFormatTable7"=38, "xlRangeAutoFormatTable8"=39, "xlRangeAutoFormatTable9"=40, "xlRangeAutoFormatTable10"=41, "xlRangeAutoFormatPTNone"=42, "xlRangeAutoFormatNone"=-4142, "xlRangeAutoFormatSimple"=-4154] ("auto format (none)")
                n77 = Get Date/Time In Seconds() -> (seconds since 1Jan1904=w197:timestamp)
                n78 = Format Date/Time String(time format string (%c)="%Y/%m/%d %H:%M:%S", seconds (now)=w197) -> (date/time string=w198:string)  [unwired: 1 in]
                n79 = Concatenate Strings("Grading Table Disc 27, Report Generated at " ("title"), w198) -> (w199:string)
                n80 = call <vilib>:"Create Report.vi"("window state (normal)"=T6."minimized", "display alerts? (F)"=FALSE, "report type"=Report_Type."Excel") -> ("report out"=w201:refnum<class "NI_report.lvclass">, "error out"=w203:errorcluster)  [unwired: 11 in]
                n81 = property on="Main Grading Table Disc 2" class="Tbl (strict)"() -> ("Value"=w204:string[][])  [unwired: 2 in, 2 out]
                n82 = call <vilib>:"Excel Easy Title.vi"("report in"=w201, "title"=w199, "start (0, 0)"=cluster{"row":i32, "column":i32} {"row"=0, "column"=2}, "font"=T4 {"font name"="Times New Roman", "font size"=24.0, "bold"=1, "italic"=0, "underline"=0, "strike through"=0, "font color"=16777216}, "error in (no error)"=w203) -> ("report out"=w200:refnum<class "NI_report.lvclass">, "error out"=w202:errorcluster)  [unwired: 8 in, 1 out]
                n83 = call-poly <vilib>:"Excel Easy Table.vi"("report in"=w200, "font"=T4 {"font name"="Times New Roman", "font size"=12.0, "bold"=0, "italic"=0, "underline"=0, "strike through"=0, "font color"=16777216}, "auto format (none)"=w188, "start (0, 0)"=cluster{"row":i32, "column":i32} {"row"=2, "column"=2}, "text data"=w204, "error in (no error)"=w202, "column headers"=string[] ["Date", "Time", "8-16mm", "10-14mm", "Disc Situation", "Control Mode", "Camera Situation", "Projector Situation"]) -> ("report out"=w184:refnum<class "NI_report.lvclass">, "error out"=w185:errorcluster)  [unwired: 4 in, 3 out]
                n84 = call-dynamic "Print Report.vi"("report in"=w184, "error in (no error)"=w185) -> ("report out"=w182:refnum<class "NI_report.lvclass">, "error out"=w183:errorcluster)  [unwired: 12 in]
                n85 = call-dynamic "Dispose Report.vi"("report in"=w182, "error in (no error)"=w183) -> ("error out"=w181:errorcluster)  [unwired: 13 in]
              }
              frame "Disc 03" {
                w212 = 1 items=["xlRangeAutoFormat3DEffects1"=13, "xlRangeAutoFormat3DEffects2"=14, "xlRangeAutoFormatAccounting1"=4, "xlRangeAutoFormatAccounting2"=5, "xlRangeAutoFormatAccounting3"=6, "xlRangeAutoFormatAccounting4"=17, "xlRangeAutoFormatClassic1"=1, "xlRangeAutoFormatClassic2"=2, "xlRangeAutoFormatClassic3"=3, "xlRangeAutoFormatColor1"=7, "xlRangeAutoFormatColor2"=8, "xlRangeAutoFormatColor3"=9, "xlRangeAutoFormatList1"=10, "xlRangeAutoFormatList2"=11, "xlRangeAutoFormatList3"=12, "xlRangeAutoFormatLocalFormat1"=15, "xlRangeAutoFormatLocalFormat2"=16, "xlRangeAutoFormatLocalFormat3"=19, "xlRangeAutoFormatLocalFormat4"=20, "xlRangeAutoFormatReport1"=21, "xlRangeAutoFormatReport2"=22, "xlRangeAutoFormatReport3"=23, "xlRangeAutoFormatReport4"=24, "xlRangeAutoFormatReport5"=25, "xlRangeAutoFormatReport6"=26, "xlRangeAutoFormatReport7"=27, "xlRangeAutoFormatReport8"=28, "xlRangeAutoFormatReport9"=29, "xlRangeAutoFormatReport10"=30, "xlRangeAutoFormatClassicPivotTable"=31, "xlRangeAutoFormatTable1"=32, "xlRangeAutoFormatTable2"=33, "xlRangeAutoFormatTable3"=34, "xlRangeAutoFormatTable4"=35, "xlRangeAutoFormatTable5"=36, "xlRangeAutoFormatTable6"=37, "xlRangeAutoFormatTable7"=38, "xlRangeAutoFormatTable8"=39, "xlRangeAutoFormatTable9"=40, "xlRangeAutoFormatTable10"=41, "xlRangeAutoFormatPTNone"=42, "xlRangeAutoFormatNone"=-4142, "xlRangeAutoFormatSimple"=-4154] ("auto format (none)")
                n86 = Get Date/Time In Seconds() -> (seconds since 1Jan1904=w221:timestamp)
                n87 = Format Date/Time String(time format string (%c)="%Y/%m/%d %H:%M:%S", seconds (now)=w221) -> (date/time string=w222:string)  [unwired: 1 in]
                n88 = Concatenate Strings("Grading Table Disc 28, Report Generated at " ("title"), w222) -> (w223:string)
                n89 = call <vilib>:"Create Report.vi"("window state (normal)"=T6."minimized", "display alerts? (F)"=FALSE, "report type"=Report_Type."Excel") -> ("report out"=w225:refnum<class "NI_report.lvclass">, "error out"=w227:errorcluster)  [unwired: 11 in]
                n90 = property on="Main Grading Table Disc 3" class="Tbl (strict)"() -> ("Value"=w228:string[][])  [unwired: 2 in, 2 out]
                n91 = call <vilib>:"Excel Easy Title.vi"("report in"=w225, "title"=w223, "start (0, 0)"=cluster{"row":i32, "column":i32} {"row"=0, "column"=2}, "font"=T4 {"font name"="Times New Roman", "font size"=24.0, "bold"=1, "italic"=0, "underline"=0, "strike through"=0, "font color"=16777216}, "error in (no error)"=w227) -> ("report out"=w224:refnum<class "NI_report.lvclass">, "error out"=w226:errorcluster)  [unwired: 8 in, 1 out]
                n92 = call-poly <vilib>:"Excel Easy Table.vi"("report in"=w224, "font"=T4 {"font name"="Times New Roman", "font size"=12.0, "bold"=0, "italic"=0, "underline"=0, "strike through"=0, "font color"=16777216}, "auto format (none)"=w212, "start (0, 0)"=cluster{"row":i32, "column":i32} {"row"=2, "column"=2}, "text data"=w228, "error in (no error)"=w226, "column headers"=string[] ["Date", "Time", "8-16mm", "10-14mm", "Disc Situation", "Control Mode", "Camera Situation", "Projector Situation"]) -> ("report out"=w208:refnum<class "NI_report.lvclass">, "error out"=w209:errorcluster)  [unwired: 4 in, 3 out]
                n93 = call-dynamic "Print Report.vi"("report in"=w208, "error in (no error)"=w209) -> ("report out"=w206:refnum<class "NI_report.lvclass">, "error out"=w207:errorcluster)  [unwired: 12 in]
                n94 = call-dynamic "Dispose Report.vi"("report in"=w206, "error in (no error)"=w207) -> ("error out"=w205:errorcluster)  [unwired: 13 in]
              }
              frame "Disc 04" {
                w236 = 1 items=["xlRangeAutoFormat3DEffects1"=13, "xlRangeAutoFormat3DEffects2"=14, "xlRangeAutoFormatAccounting1"=4, "xlRangeAutoFormatAccounting2"=5, "xlRangeAutoFormatAccounting3"=6, "xlRangeAutoFormatAccounting4"=17, "xlRangeAutoFormatClassic1"=1, "xlRangeAutoFormatClassic2"=2, "xlRangeAutoFormatClassic3"=3, "xlRangeAutoFormatColor1"=7, "xlRangeAutoFormatColor2"=8, "xlRangeAutoFormatColor3"=9, "xlRangeAutoFormatList1"=10, "xlRangeAutoFormatList2"=11, "xlRangeAutoFormatList3"=12, "xlRangeAutoFormatLocalFormat1"=15, "xlRangeAutoFormatLocalFormat2"=16, "xlRangeAutoFormatLocalFormat3"=19, "xlRangeAutoFormatLocalFormat4"=20, "xlRangeAutoFormatReport1"=21, "xlRangeAutoFormatReport2"=22, "xlRangeAutoFormatReport3"=23, "xlRangeAutoFormatReport4"=24, "xlRangeAutoFormatReport5"=25, "xlRangeAutoFormatReport6"=26, "xlRangeAutoFormatReport7"=27, "xlRangeAutoFormatReport8"=28, "xlRangeAutoFormatReport9"=29, "xlRangeAutoFormatReport10"=30, "xlRangeAutoFormatClassicPivotTable"=31, "xlRangeAutoFormatTable1"=32, "xlRangeAutoFormatTable2"=33, "xlRangeAutoFormatTable3"=34, "xlRangeAutoFormatTable4"=35, "xlRangeAutoFormatTable5"=36, "xlRangeAutoFormatTable6"=37, "xlRangeAutoFormatTable7"=38, "xlRangeAutoFormatTable8"=39, "xlRangeAutoFormatTable9"=40, "xlRangeAutoFormatTable10"=41, "xlRangeAutoFormatPTNone"=42, "xlRangeAutoFormatNone"=-4142, "xlRangeAutoFormatSimple"=-4154] ("auto format (none)")
                n95 = Get Date/Time In Seconds() -> (seconds since 1Jan1904=w245:timestamp)
                n96 = Format Date/Time String(time format string (%c)="%Y/%m/%d %H:%M:%S", seconds (now)=w245) -> (date/time string=w246:string)  [unwired: 1 in]
                n97 = Concatenate Strings("Grading Table Disc 29, Report Generated at " ("title"), w246) -> (w247:string)
                n98 = call <vilib>:"Create Report.vi"("window state (normal)"=T6."minimized", "display alerts? (F)"=FALSE, "report type"=Report_Type."Excel") -> ("report out"=w249:refnum<class "NI_report.lvclass">, "error out"=w251:errorcluster)  [unwired: 11 in]
                n99 = property on="Main Grading Table Disc 4" class="Tbl (strict)"() -> ("Value"=w252:string[][])  [unwired: 2 in, 2 out]
                n100 = call <vilib>:"Excel Easy Title.vi"("report in"=w249, "title"=w247, "start (0, 0)"=cluster{"row":i32, "column":i32} {"row"=0, "column"=2}, "font"=T4 {"font name"="Times New Roman", "font size"=24.0, "bold"=1, "italic"=0, "underline"=0, "strike through"=0, "font color"=16777216}, "error in (no error)"=w251) -> ("report out"=w248:refnum<class "NI_report.lvclass">, "error out"=w250:errorcluster)  [unwired: 8 in, 1 out]
                n101 = call-poly <vilib>:"Excel Easy Table.vi"("report in"=w248, "font"=T4 {"font name"="Times New Roman", "font size"=12.0, "bold"=0, "italic"=0, "underline"=0, "strike through"=0, "font color"=16777216}, "auto format (none)"=w236, "start (0, 0)"=cluster{"row":i32, "column":i32} {"row"=2, "column"=2}, "text data"=w252, "error in (no error)"=w250, "column headers"=string[] ["Date", "Time", "8-16mm", "10-14mm", "Disc Situation", "Control Mode", "Camera Situation", "Projector Situation"]) -> ("report out"=w232:refnum<class "NI_report.lvclass">, "error out"=w233:errorcluster)  [unwired: 4 in, 3 out]
                n102 = call-dynamic "Print Report.vi"("report in"=w232, "error in (no error)"=w233) -> ("report out"=w230:refnum<class "NI_report.lvclass">, "error out"=w231:errorcluster)  [unwired: 12 in]
                n103 = call-dynamic "Dispose Report.vi"("report in"=w230, "error in (no error)"=w231) -> ("error out"=w229:errorcluster)  [unwired: 13 in]
              }
              frame "Disc 05" {
                w260 = 1 items=["xlRangeAutoFormat3DEffects1"=13, "xlRangeAutoFormat3DEffects2"=14, "xlRangeAutoFormatAccounting1"=4, "xlRangeAutoFormatAccounting2"=5, "xlRangeAutoFormatAccounting3"=6, "xlRangeAutoFormatAccounting4"=17, "xlRangeAutoFormatClassic1"=1, "xlRangeAutoFormatClassic2"=2, "xlRangeAutoFormatClassic3"=3, "xlRangeAutoFormatColor1"=7, "xlRangeAutoFormatColor2"=8, "xlRangeAutoFormatColor3"=9, "xlRangeAutoFormatList1"=10, "xlRangeAutoFormatList2"=11, "xlRangeAutoFormatList3"=12, "xlRangeAutoFormatLocalFormat1"=15, "xlRangeAutoFormatLocalFormat2"=16, "xlRangeAutoFormatLocalFormat3"=19, "xlRangeAutoFormatLocalFormat4"=20, "xlRangeAutoFormatReport1"=21, "xlRangeAutoFormatReport2"=22, "xlRangeAutoFormatReport3"=23, "xlRangeAutoFormatReport4"=24, "xlRangeAutoFormatReport5"=25, "xlRangeAutoFormatReport6"=26, "xlRangeAutoFormatReport7"=27, "xlRangeAutoFormatReport8"=28, "xlRangeAutoFormatReport9"=29, "xlRangeAutoFormatReport10"=30, "xlRangeAutoFormatClassicPivotTable"=31, "xlRangeAutoFormatTable1"=32, "xlRangeAutoFormatTable2"=33, "xlRangeAutoFormatTable3"=34, "xlRangeAutoFormatTable4"=35, "xlRangeAutoFormatTable5"=36, "xlRangeAutoFormatTable6"=37, "xlRangeAutoFormatTable7"=38, "xlRangeAutoFormatTable8"=39, "xlRangeAutoFormatTable9"=40, "xlRangeAutoFormatTable10"=41, "xlRangeAutoFormatPTNone"=42, "xlRangeAutoFormatNone"=-4142, "xlRangeAutoFormatSimple"=-4154] ("auto format (none)")
                n104 = Get Date/Time In Seconds() -> (seconds since 1Jan1904=w269:timestamp)
                n105 = Format Date/Time String(time format string (%c)="%Y/%m/%d %H:%M:%S", seconds (now)=w269) -> (date/time string=w270:string)  [unwired: 1 in]
                n106 = Concatenate Strings("Grading Table Disc 30, Report Generated at " ("title"), w270) -> (w271:string)
                n107 = call <vilib>:"Create Report.vi"("window state (normal)"=T6."minimized", "display alerts? (F)"=FALSE, "report type"=Report_Type."Excel") -> ("report out"=w273:refnum<class "NI_report.lvclass">, "error out"=w275:errorcluster)  [unwired: 11 in]
                n108 = property on="Main Grading Table Disc 5" class="Tbl (strict)"() -> ("Value"=w276:string[][])  [unwired: 2 in, 2 out]
                n109 = call <vilib>:"Excel Easy Title.vi"("report in"=w273, "title"=w271, "start (0, 0)"=cluster{"row":i32, "column":i32} {"row"=0, "column"=0}, "font"=T4 {"font name"="Times New Roman", "font size"=24.0, "bold"=1, "italic"=0, "underline"=0, "strike through"=0, "font color"=16777216}, "error in (no error)"=w275) -> ("report out"=w272:refnum<class "NI_report.lvclass">, "error out"=w274:errorcluster)  [unwired: 8 in, 1 out]
                n110 = call-poly <vilib>:"Excel Easy Table.vi"("report in"=w272, "font"=T4 {"font name"="Times New Roman", "font size"=12.0, "bold"=0, "italic"=0, "underline"=0, "strike through"=0, "font color"=16777216}, "auto format (none)"=w260, "start (0, 0)"=cluster{"row":i32, "column":i32} {"row"=2, "column"=0}, "text data"=w276, "error in (no error)"=w274, "column headers"=string[] ["Date", "Time", "8-16mm", "10-14mm", "Disc Situation", "Control Mode", "Camera Situation", "Projector Situation"]) -> ("report out"=w256:refnum<class "NI_report.lvclass">, "error out"=w257:errorcluster)  [unwired: 4 in, 3 out]
                n111 = call-dynamic "Print Report.vi"("report in"=w256, "error in (no error)"=w257) -> ("report out"=w254:refnum<class "NI_report.lvclass">, "error out"=w255:errorcluster)  [unwired: 12 in]
                n112 = call-dynamic "Dispose Report.vi"("report in"=w254, "error in (no error)"=w255) -> ("error out"=w253:errorcluster)  [unwired: 13 in]
              }
            }
          }
          frame "Print 3" {
            w285 = 1 items=["xlRangeAutoFormat3DEffects1"=13, "xlRangeAutoFormat3DEffects2"=14, "xlRangeAutoFormatAccounting1"=4, "xlRangeAutoFormatAccounting2"=5, "xlRangeAutoFormatAccounting3"=6, "xlRangeAutoFormatAccounting4"=17, "xlRangeAutoFormatClassic1"=1, "xlRangeAutoFormatClassic2"=2, "xlRangeAutoFormatClassic3"=3, "xlRangeAutoFormatColor1"=7, "xlRangeAutoFormatColor2"=8, "xlRangeAutoFormatColor3"=9, "xlRangeAutoFormatList1"=10, "xlRangeAutoFormatList2"=11, "xlRangeAutoFormatList3"=12, "xlRangeAutoFormatLocalFormat1"=15, "xlRangeAutoFormatLocalFormat2"=16, "xlRangeAutoFormatLocalFormat3"=19, "xlRangeAutoFormatLocalFormat4"=20, "xlRangeAutoFormatReport1"=21, "xlRangeAutoFormatReport2"=22, "xlRangeAutoFormatReport3"=23, "xlRangeAutoFormatReport4"=24, "xlRangeAutoFormatReport5"=25, "xlRangeAutoFormatReport6"=26, "xlRangeAutoFormatReport7"=27, "xlRangeAutoFormatReport8"=28, "xlRangeAutoFormatReport9"=29, "xlRangeAutoFormatReport10"=30, "xlRangeAutoFormatClassicPivotTable"=31, "xlRangeAutoFormatTable1"=32, "xlRangeAutoFormatTable2"=33, "xlRangeAutoFormatTable3"=34, "xlRangeAutoFormatTable4"=35, "xlRangeAutoFormatTable5"=36, "xlRangeAutoFormatTable6"=37, "xlRangeAutoFormatTable7"=38, "xlRangeAutoFormatTable8"=39, "xlRangeAutoFormatTable9"=40, "xlRangeAutoFormatTable10"=41, "xlRangeAutoFormatPTNone"=42, "xlRangeAutoFormatNone"=-4142, "xlRangeAutoFormatSimple"=-4154] ("auto format (none)")
            n113 = call <vilib>:"Create Report.vi"("window state (normal)"=T6."minimized", "display alerts? (F)"=FALSE, "report type"=Report_Type."Excel") -> ("report out"=w293:refnum<class "NI_report.lvclass">, "error out"=w295:errorcluster)  [unwired: 11 in]
            n114 = call <vilib>:"Excel Easy Title.vi"("report in"=w293, "title"="Log Table", "start (0, 0)"=cluster{"row":i32, "column":i32} {"row"=0, "column"=0}, "font"=T4 {"font name"="Times New Roman", "font size"=24.0, "bold"=1, "italic"=0, "underline"=0, "strike through"=0, "font color"=16777216}, "error in (no error)"=w295) -> ("report out"=w292:refnum<class "NI_report.lvclass">, "error out"=w294:errorcluster)  [unwired: 8 in, 1 out]
            n115 = property on="Log Table" class="Tbl (strict)"() -> ("Value"=w296:string[][])  [unwired: 2 in, 2 out]
            n116 = call-poly <vilib>:"Excel Easy Table.vi"("report in"=w292, "font"=T4 {"font name"="Times New Roman", "font size"=12.0, "bold"=0, "italic"=0, "underline"=0, "strike through"=0, "font color"=16777216}, "auto format (none)"=w285, "start (0, 0)"=cluster{"row":i32, "column":i32} {"row"=2, "column"=0}, "text data"=w296, "error in (no error)"=w294, "column headers"=string[] ["Log Catalog", "Date", "Time", "Description"]) -> ("report out"=w281:refnum<class "NI_report.lvclass">, "error out"=w282:errorcluster)  [unwired: 4 in, 3 out]
            n117 = call-dynamic "Print Report.vi"("report in"=w281, "error in (no error)"=w282) -> ("report out"=w279:refnum<class "NI_report.lvclass">, "error out"=w280:errorcluster)  [unwired: 12 in]
            n118 = call-dynamic "Dispose Report.vi"("report in"=w279, "error in (no error)"=w280) -> ("error out"=w277:errorcluster)  [unwired: 13 in]
          }
        }
        n119 = shared-variable ".\\Maintenance.lvlib\\error_63"(w6) -> ()  [unwired: 1 in, 1 out]
      }
      event "Save 1", "Save 2", "Save 3": Mouse Down {
        n120 = event-data() -> ("CtlRef"=w299:refnum<vi>)  [unwired: 1 in, 7 out]
        n121 = property class="Bool (strict)"(reference=w299) -> ("Label.Text"=w298:string)  [unwired: 1 in, 2 out]
        n122 = case shown="\"Save 1\", Default" w298 {
          tunnel: [w300 w422 w544] -> w297
          frame "Save 1", Default {
            n123 = property on="Tab Control 2" class="TabCtl (strict)"() -> ("Value"=w301:T2)  [unwired: 2 in, 2 out]
            n124 = case shown="\"Disc 05\"" w301 {
              tunnel: [w303 w323 w343 w363 w383 w402] -> w300
              frame "Disc 01", Default {
                w316 = 1 items=["xlRangeAutoFormat3DEffects1"=13, "xlRangeAutoFormat3DEffects2"=14, "xlRangeAutoFormatAccounting1"=4, "xlRangeAutoFormatAccounting2"=5, "xlRangeAutoFormatAccounting3"=6, "xlRangeAutoFormatAccounting4"=17, "xlRangeAutoFormatClassic1"=1, "xlRangeAutoFormatClassic2"=2, "xlRangeAutoFormatClassic3"=3, "xlRangeAutoFormatColor1"=7, "xlRangeAutoFormatColor2"=8, "xlRangeAutoFormatColor3"=9, "xlRangeAutoFormatList1"=10, "xlRangeAutoFormatList2"=11, "xlRangeAutoFormatList3"=12, "xlRangeAutoFormatLocalFormat1"=15, "xlRangeAutoFormatLocalFormat2"=16, "xlRangeAutoFormatLocalFormat3"=19, "xlRangeAutoFormatLocalFormat4"=20, "xlRangeAutoFormatReport1"=21, "xlRangeAutoFormatReport2"=22, "xlRangeAutoFormatReport3"=23, "xlRangeAutoFormatReport4"=24, "xlRangeAutoFormatReport5"=25, "xlRangeAutoFormatReport6"=26, "xlRangeAutoFormatReport7"=27, "xlRangeAutoFormatReport8"=28, "xlRangeAutoFormatReport9"=29, "xlRangeAutoFormatReport10"=30, "xlRangeAutoFormatClassicPivotTable"=31, "xlRangeAutoFormatTable1"=32, "xlRangeAutoFormatTable2"=33, "xlRangeAutoFormatTable3"=34, "xlRangeAutoFormatTable4"=35, "xlRangeAutoFormatTable5"=36, "xlRangeAutoFormatTable6"=37, "xlRangeAutoFormatTable7"=38, "xlRangeAutoFormatTable8"=39, "xlRangeAutoFormatTable9"=40, "xlRangeAutoFormatTable10"=41, "xlRangeAutoFormatPTNone"=42, "xlRangeAutoFormatNone"=-4142, "xlRangeAutoFormatSimple"=-4154] ("auto format (none)")
                n125 = Get Date/Time In Seconds() -> (seconds since 1Jan1904=w305:timestamp)
                n126 = Format Date/Time String(time format string (%c)="%Y/%m/%d %H:%M:%S", seconds (now)=w305) -> (date/time string=w306:string)  [unwired: 1 in]
                n127 = Concatenate Strings("Grading Table Disc 1, Report Generated at " ("title"), w306) -> (w307:string)
                n128 = call <vilib>:"Create Report.vi"("window state (normal)"=T6."maximized", "display alerts? (F)"=TRUE, "report type"=Report_Type."Excel") -> ("report out"=w312:refnum<class "NI_report.lvclass">, "error out"=w314:errorcluster)  [unwired: 11 in]
                n129 = property on="Grading Table Disc 1" class="Tbl (strict)"() -> ("Value"=w319:string[][])  [unwired: 2 in, 2 out]
                n130 = call <vilib>:"Excel Easy Title.vi"("report in"=w312, "title"=w307, "start (0, 0)"=cluster{"row":i32, "column":i32} {"row"=0, "column"=2}, "font"=T4 {"font name"="Times New Roman", "font size"=24.0, "bold"=1, "italic"=0, "underline"=0, "strike through"=0, "font color"=16777216}, "error in (no error)"=w314) -> ("report out"=w311:refnum<class "NI_report.lvclass">, "error out"=w313:errorcluster)  [unwired: 8 in, 1 out]
                n131 = call-poly <vilib>:"Excel Easy Table.vi"("report in"=w311, "font"=T4 {"font name"="Times New Roman", "font size"=12.0, "bold"=0, "italic"=0, "underline"=0, "strike through"=0, "font color"=16777216}, "auto format (none)"=w316, "start (0, 0)"=cluster{"row":i32, "column":i32} {"row"=2, "column"=2}, "text data"=w319, "error in (no error)"=w313, "column headers"=string[] ["Date", "Time", "<6.3mm", "6.3-8mm", "8-9.5mm", "9.5-11mm", "11-12.7mm", "12.7-14mm", "14-16mm", "16mm<", "Disc Situation", "Control Mode", "Camera Situation", "Projector Situation"]) -> ("error out"=w303:errorcluster)  [unwired: 4 in, 4 out]
              }
              frame "Disc 02" {
                w325 = 1 items=["xlRangeAutoFormat3DEffects1"=13, "xlRangeAutoFormat3DEffects2"=14, "xlRangeAutoFormatAccounting1"=4, "xlRangeAutoFormatAccounting2"=5, "xlRangeAutoFormatAccounting3"=6, "xlRangeAutoFormatAccounting4"=17, "xlRangeAutoFormatClassic1"=1, "xlRangeAutoFormatClassic2"=2, "xlRangeAutoFormatClassic3"=3, "xlRangeAutoFormatColor1"=7, "xlRangeAutoFormatColor2"=8, "xlRangeAutoFormatColor3"=9, "xlRangeAutoFormatList1"=10, "xlRangeAutoFormatList2"=11, "xlRangeAutoFormatList3"=12, "xlRangeAutoFormatLocalFormat1"=15, "xlRangeAutoFormatLocalFormat2"=16, "xlRangeAutoFormatLocalFormat3"=19, "xlRangeAutoFormatLocalFormat4"=20, "xlRangeAutoFormatReport1"=21, "xlRangeAutoFormatReport2"=22, "xlRangeAutoFormatReport3"=23, "xlRangeAutoFormatReport4"=24, "xlRangeAutoFormatReport5"=25, "xlRangeAutoFormatReport6"=26, "xlRangeAutoFormatReport7"=27, "xlRangeAutoFormatReport8"=28, "xlRangeAutoFormatReport9"=29, "xlRangeAutoFormatReport10"=30, "xlRangeAutoFormatClassicPivotTable"=31, "xlRangeAutoFormatTable1"=32, "xlRangeAutoFormatTable2"=33, "xlRangeAutoFormatTable3"=34, "xlRangeAutoFormatTable4"=35, "xlRangeAutoFormatTable5"=36, "xlRangeAutoFormatTable6"=37, "xlRangeAutoFormatTable7"=38, "xlRangeAutoFormatTable8"=39, "xlRangeAutoFormatTable9"=40, "xlRangeAutoFormatTable10"=41, "xlRangeAutoFormatPTNone"=42, "xlRangeAutoFormatNone"=-4142, "xlRangeAutoFormatSimple"=-4154] ("auto format (none)")
                n132 = Get Date/Time In Seconds() -> (seconds since 1Jan1904=w334:timestamp)
                n133 = Format Date/Time String(time format string (%c)="%Y/%m/%d %H:%M:%S", seconds (now)=w334) -> (date/time string=w335:string)  [unwired: 1 in]
                n134 = Concatenate Strings("Grading Table Disc 2, Report Generated at " ("title"), w335) -> (w336:string)
                n135 = call <vilib>:"Create Report.vi"("window state (normal)"=T6."maximized", "display alerts? (F)"=TRUE, "report type"=Report_Type."Excel") -> ("report out"=w338:refnum<class "NI_report.lvclass">, "error out"=w340:errorcluster)  [unwired: 11 in]
                n136 = property on="Grading Table Disc 2" class="Tbl (strict)"() -> ("Value"=w341:string[][])  [unwired: 2 in, 2 out]
                n137 = call <vilib>:"Excel Easy Title.vi"("report in"=w338, "title"=w336, "start (0, 0)"=cluster{"row":i32, "column":i32} {"row"=0, "column"=2}, "font"=T4 {"font name"="Times New Roman", "font size"=24.0, "bold"=1, "italic"=0, "underline"=0, "strike through"=0, "font color"=16777216}, "error in (no error)"=w340) -> ("report out"=w337:refnum<class "NI_report.lvclass">, "error out"=w339:errorcluster)  [unwired: 8 in, 1 out]
                n138 = call-poly <vilib>:"Excel Easy Table.vi"("report in"=w337, "font"=T4 {"font name"="Times New Roman", "font size"=12.0, "bold"=0, "italic"=0, "underline"=0, "strike through"=0, "font color"=16777216}, "auto format (none)"=w325, "start (0, 0)"=cluster{"row":i32, "column":i32} {"row"=2, "column"=2}, "text data"=w341, "error in (no error)"=w339, "column headers"=string[] ["Date", "Time", "<6.3mm", "6.3-8mm", "8-9.5mm", "9.5-11mm", "11-12.7mm", "12.7-14mm", "14-16mm", "16mm<", "Disc Situation", "Control Mode", "Camera Situation", "Projector Situation"]) -> ("error out"=w323:errorcluster)  [unwired: 4 in, 4 out]
              }
              frame "Disc 03" {
                w345 = 1 items=["xlRangeAutoFormat3DEffects1"=13, "xlRangeAutoFormat3DEffects2"=14, "xlRangeAutoFormatAccounting1"=4, "xlRangeAutoFormatAccounting2"=5, "xlRangeAutoFormatAccounting3"=6, "xlRangeAutoFormatAccounting4"=17, "xlRangeAutoFormatClassic1"=1, "xlRangeAutoFormatClassic2"=2, "xlRangeAutoFormatClassic3"=3, "xlRangeAutoFormatColor1"=7, "xlRangeAutoFormatColor2"=8, "xlRangeAutoFormatColor3"=9, "xlRangeAutoFormatList1"=10, "xlRangeAutoFormatList2"=11, "xlRangeAutoFormatList3"=12, "xlRangeAutoFormatLocalFormat1"=15, "xlRangeAutoFormatLocalFormat2"=16, "xlRangeAutoFormatLocalFormat3"=19, "xlRangeAutoFormatLocalFormat4"=20, "xlRangeAutoFormatReport1"=21, "xlRangeAutoFormatReport2"=22, "xlRangeAutoFormatReport3"=23, "xlRangeAutoFormatReport4"=24, "xlRangeAutoFormatReport5"=25, "xlRangeAutoFormatReport6"=26, "xlRangeAutoFormatReport7"=27, "xlRangeAutoFormatReport8"=28, "xlRangeAutoFormatReport9"=29, "xlRangeAutoFormatReport10"=30, "xlRangeAutoFormatClassicPivotTable"=31, "xlRangeAutoFormatTable1"=32, "xlRangeAutoFormatTable2"=33, "xlRangeAutoFormatTable3"=34, "xlRangeAutoFormatTable4"=35, "xlRangeAutoFormatTable5"=36, "xlRangeAutoFormatTable6"=37, "xlRangeAutoFormatTable7"=38, "xlRangeAutoFormatTable8"=39, "xlRangeAutoFormatTable9"=40, "xlRangeAutoFormatTable10"=41, "xlRangeAutoFormatPTNone"=42, "xlRangeAutoFormatNone"=-4142, "xlRangeAutoFormatSimple"=-4154] ("auto format (none)")
                n139 = Get Date/Time In Seconds() -> (seconds since 1Jan1904=w354:timestamp)
                n140 = Format Date/Time String(time format string (%c)="%Y/%m/%d %H:%M:%S", seconds (now)=w354) -> (date/time string=w355:string)  [unwired: 1 in]
                n141 = Concatenate Strings("Grading Table Disc 3, Report Generated at " ("title"), w355) -> (w356:string)
                n142 = call <vilib>:"Create Report.vi"("window state (normal)"=T6."maximized", "display alerts? (F)"=TRUE, "report type"=Report_Type."Excel") -> ("report out"=w358:refnum<class "NI_report.lvclass">, "error out"=w360:errorcluster)  [unwired: 11 in]
                n143 = property on="Grading Table Disc 3" class="Tbl (strict)"() -> ("Value"=w361:string[][])  [unwired: 2 in, 2 out]
                n144 = call <vilib>:"Excel Easy Title.vi"("report in"=w358, "title"=w356, "start (0, 0)"=cluster{"row":i32, "column":i32} {"row"=0, "column"=2}, "font"=T4 {"font name"="Times New Roman", "font size"=24.0, "bold"=1, "italic"=0, "underline"=0, "strike through"=0, "font color"=16777216}, "error in (no error)"=w360) -> ("report out"=w357:refnum<class "NI_report.lvclass">, "error out"=w359:errorcluster)  [unwired: 8 in, 1 out]
                n145 = call-poly <vilib>:"Excel Easy Table.vi"("report in"=w357, "font"=T4 {"font name"="Times New Roman", "font size"=12.0, "bold"=0, "italic"=0, "underline"=0, "strike through"=0, "font color"=16777216}, "auto format (none)"=w345, "start (0, 0)"=cluster{"row":i32, "column":i32} {"row"=2, "column"=2}, "text data"=w361, "error in (no error)"=w359, "column headers"=string[] ["Date", "Time", "<6.3mm", "6.3-8mm", "8-9.5mm", "9.5-11mm", "11-12.7mm", "12.7-14mm", "14-16mm", "16mm<", "Disc Situation", "Control Mode", "Camera Situation", "Projector Situation"]) -> ("error out"=w343:errorcluster)  [unwired: 4 in, 4 out]
              }
              frame "Disc 04" {
                w365 = 1 items=["xlRangeAutoFormat3DEffects1"=13, "xlRangeAutoFormat3DEffects2"=14, "xlRangeAutoFormatAccounting1"=4, "xlRangeAutoFormatAccounting2"=5, "xlRangeAutoFormatAccounting3"=6, "xlRangeAutoFormatAccounting4"=17, "xlRangeAutoFormatClassic1"=1, "xlRangeAutoFormatClassic2"=2, "xlRangeAutoFormatClassic3"=3, "xlRangeAutoFormatColor1"=7, "xlRangeAutoFormatColor2"=8, "xlRangeAutoFormatColor3"=9, "xlRangeAutoFormatList1"=10, "xlRangeAutoFormatList2"=11, "xlRangeAutoFormatList3"=12, "xlRangeAutoFormatLocalFormat1"=15, "xlRangeAutoFormatLocalFormat2"=16, "xlRangeAutoFormatLocalFormat3"=19, "xlRangeAutoFormatLocalFormat4"=20, "xlRangeAutoFormatReport1"=21, "xlRangeAutoFormatReport2"=22, "xlRangeAutoFormatReport3"=23, "xlRangeAutoFormatReport4"=24, "xlRangeAutoFormatReport5"=25, "xlRangeAutoFormatReport6"=26, "xlRangeAutoFormatReport7"=27, "xlRangeAutoFormatReport8"=28, "xlRangeAutoFormatReport9"=29, "xlRangeAutoFormatReport10"=30, "xlRangeAutoFormatClassicPivotTable"=31, "xlRangeAutoFormatTable1"=32, "xlRangeAutoFormatTable2"=33, "xlRangeAutoFormatTable3"=34, "xlRangeAutoFormatTable4"=35, "xlRangeAutoFormatTable5"=36, "xlRangeAutoFormatTable6"=37, "xlRangeAutoFormatTable7"=38, "xlRangeAutoFormatTable8"=39, "xlRangeAutoFormatTable9"=40, "xlRangeAutoFormatTable10"=41, "xlRangeAutoFormatPTNone"=42, "xlRangeAutoFormatNone"=-4142, "xlRangeAutoFormatSimple"=-4154] ("auto format (none)")
                n146 = Get Date/Time In Seconds() -> (seconds since 1Jan1904=w374:timestamp)
                n147 = Format Date/Time String(time format string (%c)="%Y/%m/%d %H:%M:%S", seconds (now)=w374) -> (date/time string=w375:string)  [unwired: 1 in]
                n148 = Concatenate Strings("Grading Table Disc 4, Report Generated at " ("title"), w375) -> (w376:string)
                n149 = call <vilib>:"Create Report.vi"("window state (normal)"=T6."maximized", "display alerts? (F)"=TRUE, "report type"=Report_Type."Excel") -> ("report out"=w378:refnum<class "NI_report.lvclass">, "error out"=w380:errorcluster)  [unwired: 11 in]
                n150 = property on="Grading Table Disc 4" class="Tbl (strict)"() -> ("Value"=w381:string[][])  [unwired: 2 in, 2 out]
                n151 = call <vilib>:"Excel Easy Title.vi"("report in"=w378, "title"=w376, "start (0, 0)"=cluster{"row":i32, "column":i32} {"row"=0, "column"=2}, "font"=T4 {"font name"="Times New Roman", "font size"=24.0, "bold"=1, "italic"=0, "underline"=0, "strike through"=0, "font color"=16777216}, "error in (no error)"=w380) -> ("report out"=w377:refnum<class "NI_report.lvclass">, "error out"=w379:errorcluster)  [unwired: 8 in, 1 out]
                n152 = call-poly <vilib>:"Excel Easy Table.vi"("report in"=w377, "font"=T4 {"font name"="Times New Roman", "font size"=12.0, "bold"=0, "italic"=0, "underline"=0, "strike through"=0, "font color"=16777216}, "auto format (none)"=w365, "start (0, 0)"=cluster{"row":i32, "column":i32} {"row"=2, "column"=2}, "text data"=w381, "error in (no error)"=w379, "column headers"=string[] ["Date", "Time", "<6.3mm", "6.3-8mm", "8-9.5mm", "9.5-11mm", "11-12.7mm", "12.7-14mm", "14-16mm", "16mm<", "Disc Situation", "Control Mode", "Camera Situation", "Projector Situation"]) -> ("error out"=w363:errorcluster)  [unwired: 4 in, 4 out]
              }
              frame "Disc 05" {
                w385 = 1 items=["xlRangeAutoFormat3DEffects1"=13, "xlRangeAutoFormat3DEffects2"=14, "xlRangeAutoFormatAccounting1"=4, "xlRangeAutoFormatAccounting2"=5, "xlRangeAutoFormatAccounting3"=6, "xlRangeAutoFormatAccounting4"=17, "xlRangeAutoFormatClassic1"=1, "xlRangeAutoFormatClassic2"=2, "xlRangeAutoFormatClassic3"=3, "xlRangeAutoFormatColor1"=7, "xlRangeAutoFormatColor2"=8, "xlRangeAutoFormatColor3"=9, "xlRangeAutoFormatList1"=10, "xlRangeAutoFormatList2"=11, "xlRangeAutoFormatList3"=12, "xlRangeAutoFormatLocalFormat1"=15, "xlRangeAutoFormatLocalFormat2"=16, "xlRangeAutoFormatLocalFormat3"=19, "xlRangeAutoFormatLocalFormat4"=20, "xlRangeAutoFormatReport1"=21, "xlRangeAutoFormatReport2"=22, "xlRangeAutoFormatReport3"=23, "xlRangeAutoFormatReport4"=24, "xlRangeAutoFormatReport5"=25, "xlRangeAutoFormatReport6"=26, "xlRangeAutoFormatReport7"=27, "xlRangeAutoFormatReport8"=28, "xlRangeAutoFormatReport9"=29, "xlRangeAutoFormatReport10"=30, "xlRangeAutoFormatClassicPivotTable"=31, "xlRangeAutoFormatTable1"=32, "xlRangeAutoFormatTable2"=33, "xlRangeAutoFormatTable3"=34, "xlRangeAutoFormatTable4"=35, "xlRangeAutoFormatTable5"=36, "xlRangeAutoFormatTable6"=37, "xlRangeAutoFormatTable7"=38, "xlRangeAutoFormatTable8"=39, "xlRangeAutoFormatTable9"=40, "xlRangeAutoFormatTable10"=41, "xlRangeAutoFormatPTNone"=42, "xlRangeAutoFormatNone"=-4142, "xlRangeAutoFormatSimple"=-4154] ("auto format (none)")
                n153 = Get Date/Time In Seconds() -> (seconds since 1Jan1904=w394:timestamp)
                n154 = Format Date/Time String(time format string (%c)="%Y/%m/%d %H:%M:%S", seconds (now)=w394) -> (date/time string=w395:string)  [unwired: 1 in]
                n155 = Concatenate Strings("Grading Table Disc 5, Report Generated at " ("title"), w395) -> (w396:string)
                n156 = call <vilib>:"Create Report.vi"("window state (normal)"=T6."maximized", "display alerts? (F)"=TRUE, "report type"=Report_Type."Excel") -> ("report out"=w398:refnum<class "NI_report.lvclass">, "error out"=w400:errorcluster)  [unwired: 11 in]
                n157 = property on="Grading Table Disc 5" class="Tbl (strict)"() -> ("Value"=w401:string[][])  [unwired: 2 in, 2 out]
                n158 = call <vilib>:"Excel Easy Title.vi"("report in"=w398, "title"=w396, "start (0, 0)"=cluster{"row":i32, "column":i32} {"row"=0, "column"=2}, "font"=T4 {"font name"="Times New Roman", "font size"=24.0, "bold"=1, "italic"=0, "underline"=0, "strike through"=0, "font color"=16777216}, "error in (no error)"=w400) -> ("report out"=w397:refnum<class "NI_report.lvclass">, "error out"=w399:errorcluster)  [unwired: 8 in, 1 out]
                n159 = call-poly <vilib>:"Excel Easy Table.vi"("report in"=w397, "font"=T4 {"font name"="Times New Roman", "font size"=12.0, "bold"=0, "italic"=0, "underline"=0, "strike through"=0, "font color"=16777216}, "auto format (none)"=w385, "start (0, 0)"=cluster{"row":i32, "column":i32} {"row"=2, "column"=2}, "text data"=w401, "error in (no error)"=w399, "column headers"=string[] ["Date", "Time", "<6.3mm", "6.3-8mm", "8-9.5mm", "9.5-11mm", "11-12.7mm", "12.7-14mm", "14-16mm", "16mm<", "Disc Situation", "Control Mode", "Camera Situation", "Projector Situation"]) -> ("error out"=w383:errorcluster)  [unwired: 4 in, 4 out]
              }
              frame "Disc 06" {
                w403 = 1 items=["xlRangeAutoFormat3DEffects1"=13, "xlRangeAutoFormat3DEffects2"=14, "xlRangeAutoFormatAccounting1"=4, "xlRangeAutoFormatAccounting2"=5, "xlRangeAutoFormatAccounting3"=6, "xlRangeAutoFormatAccounting4"=17, "xlRangeAutoFormatClassic1"=1, "xlRangeAutoFormatClassic2"=2, "xlRangeAutoFormatClassic3"=3, "xlRangeAutoFormatColor1"=7, "xlRangeAutoFormatColor2"=8, "xlRangeAutoFormatColor3"=9, "xlRangeAutoFormatList1"=10, "xlRangeAutoFormatList2"=11, "xlRangeAutoFormatList3"=12, "xlRangeAutoFormatLocalFormat1"=15, "xlRangeAutoFormatLocalFormat2"=16, "xlRangeAutoFormatLocalFormat3"=19, "xlRangeAutoFormatLocalFormat4"=20, "xlRangeAutoFormatReport1"=21, "xlRangeAutoFormatReport2"=22, "xlRangeAutoFormatReport3"=23, "xlRangeAutoFormatReport4"=24, "xlRangeAutoFormatReport5"=25, "xlRangeAutoFormatReport6"=26, "xlRangeAutoFormatReport7"=27, "xlRangeAutoFormatReport8"=28, "xlRangeAutoFormatReport9"=29, "xlRangeAutoFormatReport10"=30, "xlRangeAutoFormatClassicPivotTable"=31, "xlRangeAutoFormatTable1"=32, "xlRangeAutoFormatTable2"=33, "xlRangeAutoFormatTable3"=34, "xlRangeAutoFormatTable4"=35, "xlRangeAutoFormatTable5"=36, "xlRangeAutoFormatTable6"=37, "xlRangeAutoFormatTable7"=38, "xlRangeAutoFormatTable8"=39, "xlRangeAutoFormatTable9"=40, "xlRangeAutoFormatTable10"=41, "xlRangeAutoFormatPTNone"=42, "xlRangeAutoFormatNone"=-4142, "xlRangeAutoFormatSimple"=-4154] ("auto format (none)")
                n160 = Get Date/Time In Seconds() -> (seconds since 1Jan1904=w414:timestamp)
                n161 = Format Date/Time String(time format string (%c)="%Y/%m/%d %H:%M:%S", seconds (now)=w414) -> (date/time string=w415:string)  [unwired: 1 in]
                n162 = Concatenate Strings("Grading Table Disc 6, Report Generated at " ("title"), w415) -> (w416:string)
                n163 = call <vilib>:"Create Report.vi"("window state (normal)"=T6."maximized", "display alerts? (F)"=TRUE, "report type"=Report_Type."Excel") -> ("report out"=w418:refnum<class "NI_report.lvclass">, "error out"=w420:errorcluster)  [unwired: 11 in]
                n164 = property on="Grading Table Disc 6" class="Tbl (strict)"() -> ("Value"=w421:string[][])  [unwired: 2 in, 2 out]
                n165 = call <vilib>:"Excel Easy Title.vi"("report in"=w418, "title"=w416, "start (0, 0)"=cluster{"row":i32, "column":i32} {"row"=0, "column"=2}, "font"=T4 {"font name"="Times New Roman", "font size"=24.0, "bold"=1, "italic"=0, "underline"=0, "strike through"=0, "font color"=16777216}, "error in (no error)"=w420) -> ("report out"=w417:refnum<class "NI_report.lvclass">, "error out"=w419:errorcluster)  [unwired: 8 in, 1 out]
                n166 = call-poly <vilib>:"Excel Easy Table.vi"("report in"=w417, "font"=T4 {"font name"="Times New Roman", "font size"=12.0, "bold"=0, "italic"=0, "underline"=0, "strike through"=0, "font color"=16777216}, "auto format (none)"=w403, "start (0, 0)"=cluster{"row":i32, "column":i32} {"row"=2, "column"=2}, "text data"=w421, "error in (no error)"=w419, "column headers"=string[] ["Date", "Time", "<6.3mm", "6.3-8mm", "8-9.5mm", "9.5-11mm", "11-12.7mm", "12.7-14mm", "14-16mm", "16mm<", "Disc Situation", "Control Mode", "Camera Situation", "Projector Situation"]) -> ("error out"=w402:errorcluster)  [unwired: 4 in, 4 out]
              }
            }
          }
          frame "Save 2" {
            n167 = property on="Tab Control 3" class="TabCtl (strict)"() -> ("Value"=w423:T2)  [unwired: 2 in, 2 out]
            n168 = case shown="\"Disc 06\"" w423 {
              tunnel: [w424 w444 w464 w484 w504 w524] -> w422
              frame "Disc 01", Default {
                w438 = 1 items=["xlRangeAutoFormat3DEffects1"=13, "xlRangeAutoFormat3DEffects2"=14, "xlRangeAutoFormatAccounting1"=4, "xlRangeAutoFormatAccounting2"=5, "xlRangeAutoFormatAccounting3"=6, "xlRangeAutoFormatAccounting4"=17, "xlRangeAutoFormatClassic1"=1, "xlRangeAutoFormatClassic2"=2, "xlRangeAutoFormatClassic3"=3, "xlRangeAutoFormatColor1"=7, "xlRangeAutoFormatColor2"=8, "xlRangeAutoFormatColor3"=9, "xlRangeAutoFormatList1"=10, "xlRangeAutoFormatList2"=11, "xlRangeAutoFormatList3"=12, "xlRangeAutoFormatLocalFormat1"=15, "xlRangeAutoFormatLocalFormat2"=16, "xlRangeAutoFormatLocalFormat3"=19, "xlRangeAutoFormatLocalFormat4"=20, "xlRangeAutoFormatReport1"=21, "xlRangeAutoFormatReport2"=22, "xlRangeAutoFormatReport3"=23, "xlRangeAutoFormatReport4"=24, "xlRangeAutoFormatReport5"=25, "xlRangeAutoFormatReport6"=26, "xlRangeAutoFormatReport7"=27, "xlRangeAutoFormatReport8"=28, "xlRangeAutoFormatReport9"=29, "xlRangeAutoFormatReport10"=30, "xlRangeAutoFormatClassicPivotTable"=31, "xlRangeAutoFormatTable1"=32, "xlRangeAutoFormatTable2"=33, "xlRangeAutoFormatTable3"=34, "xlRangeAutoFormatTable4"=35, "xlRangeAutoFormatTable5"=36, "xlRangeAutoFormatTable6"=37, "xlRangeAutoFormatTable7"=38, "xlRangeAutoFormatTable8"=39, "xlRangeAutoFormatTable9"=40, "xlRangeAutoFormatTable10"=41, "xlRangeAutoFormatPTNone"=42, "xlRangeAutoFormatNone"=-4142, "xlRangeAutoFormatSimple"=-4154] ("auto format (none)")
                n169 = Get Date/Time In Seconds() -> (seconds since 1Jan1904=w427:timestamp)
                n170 = Format Date/Time String(time format string (%c)="%Y/%m/%d %H:%M:%S", seconds (now)=w427) -> (date/time string=w428:string)  [unwired: 1 in]
                n171 = Concatenate Strings("Grading Table Disc 1, Report Generated at " ("title"), w428) -> (w429:string)
                n172 = call <vilib>:"Create Report.vi"("window state (normal)"=T6."maximized", "display alerts? (F)"=TRUE, "report type"=Report_Type."Excel") -> ("report out"=w434:refnum<class "NI_report.lvclass">, "error out"=w436:errorcluster)  [unwired: 11 in]
                n173 = property on="Main Grading Table Disc 1" class="Tbl (strict)"() -> ("Value"=w441:string[][])  [unwired: 2 in, 2 out]
                n174 = call <vilib>:"Excel Easy Title.vi"("report in"=w434, "title"=w429, "start (0, 0)"=cluster{"row":i32, "column":i32} {"row"=0, "column"=2}, "font"=T4 {"font name"="Times New Roman", "font size"=24.0, "bold"=1, "italic"=0, "underline"=0, "strike through"=0, "font color"=16777216}, "error in (no error)"=w436) -> ("report out"=w433:refnum<class "NI_report.lvclass">, "error out"=w435:errorcluster)  [unwired: 8 in, 1 out]
                n175 = call-poly <vilib>:"Excel Easy Table.vi"("report in"=w433, "font"=T4 {"font name"="Times New Roman", "font size"=12.0, "bold"=0, "italic"=0, "underline"=0, "strike through"=0, "font color"=16777216}, "auto format (none)"=w438, "start (0, 0)"=cluster{"row":i32, "column":i32} {"row"=2, "column"=2}, "text data"=w441, "error in (no error)"=w435, "column headers"=string[] ["Date", "Time", "8-16mm", "10-14mm", "Disc Situation", "Control Mode", "Camera Situation", "Projector Situation"]) -> ("error out"=w424:errorcluster)  [unwired: 4 in, 4 out]
              }
              frame "Disc 02" {
                w447 = 1 items=["xlRangeAutoFormat3DEffects1"=13, "xlRangeAutoFormat3DEffects2"=14, "xlRangeAutoFormatAccounting1"=4, "xlRangeAutoFormatAccounting2"=5, "xlRangeAutoFormatAccounting3"=6, "xlRangeAutoFormatAccounting4"=17, "xlRangeAutoFormatClassic1"=1, "xlRangeAutoFormatClassic2"=2, "xlRangeAutoFormatClassic3"=3, "xlRangeAutoFormatColor1"=7, "xlRangeAutoFormatColor2"=8, "xlRangeAutoFormatColor3"=9, "xlRangeAutoFormatList1"=10, "xlRangeAutoFormatList2"=11, "xlRangeAutoFormatList3"=12, "xlRangeAutoFormatLocalFormat1"=15, "xlRangeAutoFormatLocalFormat2"=16, "xlRangeAutoFormatLocalFormat3"=19, "xlRangeAutoFormatLocalFormat4"=20, "xlRangeAutoFormatReport1"=21, "xlRangeAutoFormatReport2"=22, "xlRangeAutoFormatReport3"=23, "xlRangeAutoFormatReport4"=24, "xlRangeAutoFormatReport5"=25, "xlRangeAutoFormatReport6"=26, "xlRangeAutoFormatReport7"=27, "xlRangeAutoFormatReport8"=28, "xlRangeAutoFormatReport9"=29, "xlRangeAutoFormatReport10"=30, "xlRangeAutoFormatClassicPivotTable"=31, "xlRangeAutoFormatTable1"=32, "xlRangeAutoFormatTable2"=33, "xlRangeAutoFormatTable3"=34, "xlRangeAutoFormatTable4"=35, "xlRangeAutoFormatTable5"=36, "xlRangeAutoFormatTable6"=37, "xlRangeAutoFormatTable7"=38, "xlRangeAutoFormatTable8"=39, "xlRangeAutoFormatTable9"=40, "xlRangeAutoFormatTable10"=41, "xlRangeAutoFormatPTNone"=42, "xlRangeAutoFormatNone"=-4142, "xlRangeAutoFormatSimple"=-4154] ("auto format (none)")
                n176 = Get Date/Time In Seconds() -> (seconds since 1Jan1904=w456:timestamp)
                n177 = Format Date/Time String(time format string (%c)="%Y/%m/%d %H:%M:%S", seconds (now)=w456) -> (date/time string=w457:string)  [unwired: 1 in]
                n178 = Concatenate Strings("Grading Table Disc 2, Report Generated at " ("title"), w457) -> (w458:string)
                n179 = call <vilib>:"Create Report.vi"("window state (normal)"=T6."maximized", "display alerts? (F)"=TRUE, "report type"=Report_Type."Excel") -> ("report out"=w460:refnum<class "NI_report.lvclass">, "error out"=w462:errorcluster)  [unwired: 11 in]
                n180 = property on="Main Grading Table Disc 2" class="Tbl (strict)"() -> ("Value"=w463:string[][])  [unwired: 2 in, 2 out]
                n181 = call <vilib>:"Excel Easy Title.vi"("report in"=w460, "title"=w458, "start (0, 0)"=cluster{"row":i32, "column":i32} {"row"=0, "column"=2}, "font"=T4 {"font name"="Times New Roman", "font size"=24.0, "bold"=1, "italic"=0, "underline"=0, "strike through"=0, "font color"=16777216}, "error in (no error)"=w462) -> ("report out"=w459:refnum<class "NI_report.lvclass">, "error out"=w461:errorcluster)  [unwired: 8 in, 1 out]
                n182 = call-poly <vilib>:"Excel Easy Table.vi"("report in"=w459, "font"=T4 {"font name"="Times New Roman", "font size"=12.0, "bold"=0, "italic"=0, "underline"=0, "strike through"=0, "font color"=16777216}, "auto format (none)"=w447, "start (0, 0)"=cluster{"row":i32, "column":i32} {"row"=2, "column"=2}, "text data"=w463, "error in (no error)"=w461, "column headers"=string[] ["Date", "Time", "8-16mm", "10-14mm", "Disc Situation", "Control Mode", "Camera Situation", "Projector Situation"]) -> ("error out"=w444:errorcluster)  [unwired: 4 in, 4 out]
              }
              frame "Disc 03" {
                w467 = 1 items=["xlRangeAutoFormat3DEffects1"=13, "xlRangeAutoFormat3DEffects2"=14, "xlRangeAutoFormatAccounting1"=4, "xlRangeAutoFormatAccounting2"=5, "xlRangeAutoFormatAccounting3"=6, "xlRangeAutoFormatAccounting4"=17, "xlRangeAutoFormatClassic1"=1, "xlRangeAutoFormatClassic2"=2, "xlRangeAutoFormatClassic3"=3, "xlRangeAutoFormatColor1"=7, "xlRangeAutoFormatColor2"=8, "xlRangeAutoFormatColor3"=9, "xlRangeAutoFormatList1"=10, "xlRangeAutoFormatList2"=11, "xlRangeAutoFormatList3"=12, "xlRangeAutoFormatLocalFormat1"=15, "xlRangeAutoFormatLocalFormat2"=16, "xlRangeAutoFormatLocalFormat3"=19, "xlRangeAutoFormatLocalFormat4"=20, "xlRangeAutoFormatReport1"=21, "xlRangeAutoFormatReport2"=22, "xlRangeAutoFormatReport3"=23, "xlRangeAutoFormatReport4"=24, "xlRangeAutoFormatReport5"=25, "xlRangeAutoFormatReport6"=26, "xlRangeAutoFormatReport7"=27, "xlRangeAutoFormatReport8"=28, "xlRangeAutoFormatReport9"=29, "xlRangeAutoFormatReport10"=30, "xlRangeAutoFormatClassicPivotTable"=31, "xlRangeAutoFormatTable1"=32, "xlRangeAutoFormatTable2"=33, "xlRangeAutoFormatTable3"=34, "xlRangeAutoFormatTable4"=35, "xlRangeAutoFormatTable5"=36, "xlRangeAutoFormatTable6"=37, "xlRangeAutoFormatTable7"=38, "xlRangeAutoFormatTable8"=39, "xlRangeAutoFormatTable9"=40, "xlRangeAutoFormatTable10"=41, "xlRangeAutoFormatPTNone"=42, "xlRangeAutoFormatNone"=-4142, "xlRangeAutoFormatSimple"=-4154] ("auto format (none)")
                n183 = Get Date/Time In Seconds() -> (seconds since 1Jan1904=w476:timestamp)
                n184 = Format Date/Time String(time format string (%c)="%Y/%m/%d %H:%M:%S", seconds (now)=w476) -> (date/time string=w477:string)  [unwired: 1 in]
                n185 = Concatenate Strings("Grading Table Disc 3, Report Generated at " ("title"), w477) -> (w478:string)
                n186 = call <vilib>:"Create Report.vi"("window state (normal)"=T6."maximized", "display alerts? (F)"=TRUE, "report type"=Report_Type."Excel") -> ("report out"=w480:refnum<class "NI_report.lvclass">, "error out"=w482:errorcluster)  [unwired: 11 in]
                n187 = property on="Main Grading Table Disc 3" class="Tbl (strict)"() -> ("Value"=w483:string[][])  [unwired: 2 in, 2 out]
                n188 = call <vilib>:"Excel Easy Title.vi"("report in"=w480, "title"=w478, "start (0, 0)"=cluster{"row":i32, "column":i32} {"row"=0, "column"=2}, "font"=T4 {"font name"="Times New Roman", "font size"=24.0, "bold"=1, "italic"=0, "underline"=0, "strike through"=0, "font color"=16777216}, "error in (no error)"=w482) -> ("report out"=w479:refnum<class "NI_report.lvclass">, "error out"=w481:errorcluster)  [unwired: 8 in, 1 out]
                n189 = call-poly <vilib>:"Excel Easy Table.vi"("report in"=w479, "font"=T4 {"font name"="Times New Roman", "font size"=12.0, "bold"=0, "italic"=0, "underline"=0, "strike through"=0, "font color"=16777216}, "auto format (none)"=w467, "start (0, 0)"=cluster{"row":i32, "column":i32} {"row"=2, "column"=2}, "text data"=w483, "error in (no error)"=w481, "column headers"=string[] ["Date", "Time", "8-16mm", "10-14mm", "Disc Situation", "Control Mode", "Camera Situation", "Projector Situation"]) -> ("error out"=w464:errorcluster)  [unwired: 4 in, 4 out]
              }
              frame "Disc 04" {
                w487 = 1 items=["xlRangeAutoFormat3DEffects1"=13, "xlRangeAutoFormat3DEffects2"=14, "xlRangeAutoFormatAccounting1"=4, "xlRangeAutoFormatAccounting2"=5, "xlRangeAutoFormatAccounting3"=6, "xlRangeAutoFormatAccounting4"=17, "xlRangeAutoFormatClassic1"=1, "xlRangeAutoFormatClassic2"=2, "xlRangeAutoFormatClassic3"=3, "xlRangeAutoFormatColor1"=7, "xlRangeAutoFormatColor2"=8, "xlRangeAutoFormatColor3"=9, "xlRangeAutoFormatList1"=10, "xlRangeAutoFormatList2"=11, "xlRangeAutoFormatList3"=12, "xlRangeAutoFormatLocalFormat1"=15, "xlRangeAutoFormatLocalFormat2"=16, "xlRangeAutoFormatLocalFormat3"=19, "xlRangeAutoFormatLocalFormat4"=20, "xlRangeAutoFormatReport1"=21, "xlRangeAutoFormatReport2"=22, "xlRangeAutoFormatReport3"=23, "xlRangeAutoFormatReport4"=24, "xlRangeAutoFormatReport5"=25, "xlRangeAutoFormatReport6"=26, "xlRangeAutoFormatReport7"=27, "xlRangeAutoFormatReport8"=28, "xlRangeAutoFormatReport9"=29, "xlRangeAutoFormatReport10"=30, "xlRangeAutoFormatClassicPivotTable"=31, "xlRangeAutoFormatTable1"=32, "xlRangeAutoFormatTable2"=33, "xlRangeAutoFormatTable3"=34, "xlRangeAutoFormatTable4"=35, "xlRangeAutoFormatTable5"=36, "xlRangeAutoFormatTable6"=37, "xlRangeAutoFormatTable7"=38, "xlRangeAutoFormatTable8"=39, "xlRangeAutoFormatTable9"=40, "xlRangeAutoFormatTable10"=41, "xlRangeAutoFormatPTNone"=42, "xlRangeAutoFormatNone"=-4142, "xlRangeAutoFormatSimple"=-4154] ("auto format (none)")
                n190 = Get Date/Time In Seconds() -> (seconds since 1Jan1904=w496:timestamp)
                n191 = Format Date/Time String(time format string (%c)="%Y/%m/%d %H:%M:%S", seconds (now)=w496) -> (date/time string=w497:string)  [unwired: 1 in]
                n192 = Concatenate Strings("Grading Table Disc 4, Report Generated at " ("title"), w497) -> (w498:string)
                n193 = call <vilib>:"Create Report.vi"("window state (normal)"=T6."maximized", "display alerts? (F)"=TRUE, "report type"=Report_Type."Excel") -> ("report out"=w500:refnum<class "NI_report.lvclass">, "error out"=w502:errorcluster)  [unwired: 11 in]
                n194 = property on="Main Grading Table Disc 4" class="Tbl (strict)"() -> ("Value"=w503:string[][])  [unwired: 2 in, 2 out]
                n195 = call <vilib>:"Excel Easy Title.vi"("report in"=w500, "title"=w498, "start (0, 0)"=cluster{"row":i32, "column":i32} {"row"=0, "column"=2}, "font"=T4 {"font name"="Times New Roman", "font size"=24.0, "bold"=1, "italic"=0, "underline"=0, "strike through"=0, "font color"=16777216}, "error in (no error)"=w502) -> ("report out"=w499:refnum<class "NI_report.lvclass">, "error out"=w501:errorcluster)  [unwired: 8 in, 1 out]
                n196 = call-poly <vilib>:"Excel Easy Table.vi"("report in"=w499, "font"=T4 {"font name"="Times New Roman", "font size"=12.0, "bold"=0, "italic"=0, "underline"=0, "strike through"=0, "font color"=16777216}, "auto format (none)"=w487, "start (0, 0)"=cluster{"row":i32, "column":i32} {"row"=2, "column"=2}, "text data"=w503, "error in (no error)"=w501, "column headers"=string[] ["Date", "Time", "8-16mm", "10-14mm", "Disc Situation", "Control Mode", "Camera Situation", "Projector Situation"]) -> ("error out"=w484:errorcluster)  [unwired: 4 in, 4 out]
              }
              frame "Disc 05" {
                w507 = 1 items=["xlRangeAutoFormat3DEffects1"=13, "xlRangeAutoFormat3DEffects2"=14, "xlRangeAutoFormatAccounting1"=4, "xlRangeAutoFormatAccounting2"=5, "xlRangeAutoFormatAccounting3"=6, "xlRangeAutoFormatAccounting4"=17, "xlRangeAutoFormatClassic1"=1, "xlRangeAutoFormatClassic2"=2, "xlRangeAutoFormatClassic3"=3, "xlRangeAutoFormatColor1"=7, "xlRangeAutoFormatColor2"=8, "xlRangeAutoFormatColor3"=9, "xlRangeAutoFormatList1"=10, "xlRangeAutoFormatList2"=11, "xlRangeAutoFormatList3"=12, "xlRangeAutoFormatLocalFormat1"=15, "xlRangeAutoFormatLocalFormat2"=16, "xlRangeAutoFormatLocalFormat3"=19, "xlRangeAutoFormatLocalFormat4"=20, "xlRangeAutoFormatReport1"=21, "xlRangeAutoFormatReport2"=22, "xlRangeAutoFormatReport3"=23, "xlRangeAutoFormatReport4"=24, "xlRangeAutoFormatReport5"=25, "xlRangeAutoFormatReport6"=26, "xlRangeAutoFormatReport7"=27, "xlRangeAutoFormatReport8"=28, "xlRangeAutoFormatReport9"=29, "xlRangeAutoFormatReport10"=30, "xlRangeAutoFormatClassicPivotTable"=31, "xlRangeAutoFormatTable1"=32, "xlRangeAutoFormatTable2"=33, "xlRangeAutoFormatTable3"=34, "xlRangeAutoFormatTable4"=35, "xlRangeAutoFormatTable5"=36, "xlRangeAutoFormatTable6"=37, "xlRangeAutoFormatTable7"=38, "xlRangeAutoFormatTable8"=39, "xlRangeAutoFormatTable9"=40, "xlRangeAutoFormatTable10"=41, "xlRangeAutoFormatPTNone"=42, "xlRangeAutoFormatNone"=-4142, "xlRangeAutoFormatSimple"=-4154] ("auto format (none)")
                n197 = Get Date/Time In Seconds() -> (seconds since 1Jan1904=w516:timestamp)
                n198 = Format Date/Time String(time format string (%c)="%Y/%m/%d %H:%M:%S", seconds (now)=w516) -> (date/time string=w517:string)  [unwired: 1 in]
                n199 = Concatenate Strings("Grading Table Disc 5, Report Generated at " ("title"), w517) -> (w518:string)
                n200 = call <vilib>:"Create Report.vi"("window state (normal)"=T6."maximized", "display alerts? (F)"=TRUE, "report type"=Report_Type."Excel") -> ("report out"=w520:refnum<class "NI_report.lvclass">, "error out"=w522:errorcluster)  [unwired: 11 in]
                n201 = property on="Main Grading Table Disc 5" class="Tbl (strict)"() -> ("Value"=w523:string[][])  [unwired: 2 in, 2 out]
                n202 = call <vilib>:"Excel Easy Title.vi"("report in"=w520, "title"=w518, "start (0, 0)"=cluster{"row":i32, "column":i32} {"row"=0, "column"=2}, "font"=T4 {"font name"="Times New Roman", "font size"=24.0, "bold"=1, "italic"=0, "underline"=0, "strike through"=0, "font color"=16777216}, "error in (no error)"=w522) -> ("report out"=w519:refnum<class "NI_report.lvclass">, "error out"=w521:errorcluster)  [unwired: 8 in, 1 out]
                n203 = call-poly <vilib>:"Excel Easy Table.vi"("report in"=w519, "font"=T4 {"font name"="Times New Roman", "font size"=12.0, "bold"=0, "italic"=0, "underline"=0, "strike through"=0, "font color"=16777216}, "auto format (none)"=w507, "start (0, 0)"=cluster{"row":i32, "column":i32} {"row"=2, "column"=2}, "text data"=w523, "error in (no error)"=w521, "column headers"=string[] ["Date", "Time", "8-16mm", "10-14mm", "Disc Situation", "Control Mode", "Camera Situation", "Projector Situation"]) -> ("error out"=w504:errorcluster)  [unwired: 4 in, 4 out]
              }
              frame "Disc 06" {
                w527 = 1 items=["xlRangeAutoFormat3DEffects1"=13, "xlRangeAutoFormat3DEffects2"=14, "xlRangeAutoFormatAccounting1"=4, "xlRangeAutoFormatAccounting2"=5, "xlRangeAutoFormatAccounting3"=6, "xlRangeAutoFormatAccounting4"=17, "xlRangeAutoFormatClassic1"=1, "xlRangeAutoFormatClassic2"=2, "xlRangeAutoFormatClassic3"=3, "xlRangeAutoFormatColor1"=7, "xlRangeAutoFormatColor2"=8, "xlRangeAutoFormatColor3"=9, "xlRangeAutoFormatList1"=10, "xlRangeAutoFormatList2"=11, "xlRangeAutoFormatList3"=12, "xlRangeAutoFormatLocalFormat1"=15, "xlRangeAutoFormatLocalFormat2"=16, "xlRangeAutoFormatLocalFormat3"=19, "xlRangeAutoFormatLocalFormat4"=20, "xlRangeAutoFormatReport1"=21, "xlRangeAutoFormatReport2"=22, "xlRangeAutoFormatReport3"=23, "xlRangeAutoFormatReport4"=24, "xlRangeAutoFormatReport5"=25, "xlRangeAutoFormatReport6"=26, "xlRangeAutoFormatReport7"=27, "xlRangeAutoFormatReport8"=28, "xlRangeAutoFormatReport9"=29, "xlRangeAutoFormatReport10"=30, "xlRangeAutoFormatClassicPivotTable"=31, "xlRangeAutoFormatTable1"=32, "xlRangeAutoFormatTable2"=33, "xlRangeAutoFormatTable3"=34, "xlRangeAutoFormatTable4"=35, "xlRangeAutoFormatTable5"=36, "xlRangeAutoFormatTable6"=37, "xlRangeAutoFormatTable7"=38, "xlRangeAutoFormatTable8"=39, "xlRangeAutoFormatTable9"=40, "xlRangeAutoFormatTable10"=41, "xlRangeAutoFormatPTNone"=42, "xlRangeAutoFormatNone"=-4142, "xlRangeAutoFormatSimple"=-4154] ("auto format (none)")
                n204 = Get Date/Time In Seconds() -> (seconds since 1Jan1904=w536:timestamp)
                n205 = Format Date/Time String(time format string (%c)="%Y/%m/%d %H:%M:%S", seconds (now)=w536) -> (date/time string=w537:string)  [unwired: 1 in]
                n206 = Concatenate Strings("Grading Table Disc 6, Report Generated at " ("title"), w537) -> (w538:string)
                n207 = call <vilib>:"Create Report.vi"("window state (normal)"=T6."maximized", "display alerts? (F)"=TRUE, "report type"=Report_Type."Excel") -> ("report out"=w540:refnum<class "NI_report.lvclass">, "error out"=w542:errorcluster)  [unwired: 11 in]
                n208 = property on="Main Grading Table Disc 6" class="Tbl (strict)"() -> ("Value"=w543:string[][])  [unwired: 2 in, 2 out]
                n209 = call <vilib>:"Excel Easy Title.vi"("report in"=w540, "title"=w538, "start (0, 0)"=cluster{"row":i32, "column":i32} {"row"=0, "column"=2}, "font"=T4 {"font name"="Times New Roman", "font size"=24.0, "bold"=1, "italic"=0, "underline"=0, "strike through"=0, "font color"=16777216}, "error in (no error)"=w542) -> ("report out"=w539:refnum<class "NI_report.lvclass">, "error out"=w541:errorcluster)  [unwired: 8 in, 1 out]
                n210 = call-poly <vilib>:"Excel Easy Table.vi"("report in"=w539, "font"=T4 {"font name"="Times New Roman", "font size"=12.0, "bold"=0, "italic"=0, "underline"=0, "strike through"=0, "font color"=16777216}, "auto format (none)"=w527, "start (0, 0)"=cluster{"row":i32, "column":i32} {"row"=2, "column"=2}, "text data"=w543, "error in (no error)"=w541, "column headers"=string[] ["Date", "Time", "8-16mm", "10-14mm", "Disc Situation", "Control Mode", "Camera Situation", "Projector Situation"]) -> ("error out"=w524:errorcluster)  [unwired: 4 in, 4 out]
              }
            }
          }
          frame "Save 3" {
            w547 = 1 items=["xlRangeAutoFormat3DEffects1"=13, "xlRangeAutoFormat3DEffects2"=14, "xlRangeAutoFormatAccounting1"=4, "xlRangeAutoFormatAccounting2"=5, "xlRangeAutoFormatAccounting3"=6, "xlRangeAutoFormatAccounting4"=17, "xlRangeAutoFormatClassic1"=1, "xlRangeAutoFormatClassic2"=2, "xlRangeAutoFormatClassic3"=3, "xlRangeAutoFormatColor1"=7, "xlRangeAutoFormatColor2"=8, "xlRangeAutoFormatColor3"=9, "xlRangeAutoFormatList1"=10, "xlRangeAutoFormatList2"=11, "xlRangeAutoFormatList3"=12, "xlRangeAutoFormatLocalFormat1"=15, "xlRangeAutoFormatLocalFormat2"=16, "xlRangeAutoFormatLocalFormat3"=19, "xlRangeAutoFormatLocalFormat4"=20, "xlRangeAutoFormatReport1"=21, "xlRangeAutoFormatReport2"=22, "xlRangeAutoFormatReport3"=23, "xlRangeAutoFormatReport4"=24, "xlRangeAutoFormatReport5"=25, "xlRangeAutoFormatReport6"=26, "xlRangeAutoFormatReport7"=27, "xlRangeAutoFormatReport8"=28, "xlRangeAutoFormatReport9"=29, "xlRangeAutoFormatReport10"=30, "xlRangeAutoFormatClassicPivotTable"=31, "xlRangeAutoFormatTable1"=32, "xlRangeAutoFormatTable2"=33, "xlRangeAutoFormatTable3"=34, "xlRangeAutoFormatTable4"=35, "xlRangeAutoFormatTable5"=36, "xlRangeAutoFormatTable6"=37, "xlRangeAutoFormatTable7"=38, "xlRangeAutoFormatTable8"=39, "xlRangeAutoFormatTable9"=40, "xlRangeAutoFormatTable10"=41, "xlRangeAutoFormatPTNone"=42, "xlRangeAutoFormatNone"=-4142, "xlRangeAutoFormatSimple"=-4154] ("auto format (none)")
            n211 = Get Date/Time In Seconds() -> (seconds since 1Jan1904=w556:timestamp)
            n212 = Format Date/Time String(time format string (%c)="%Y/%m/%d %H:%M:%S", seconds (now)=w556) -> (date/time string=w557:string)  [unwired: 1 in]
            n213 = Concatenate Strings("Log Table, Report Generated at " ("title"), w557) -> (w558:string)
            n214 = call <vilib>:"Create Report.vi"("window state (normal)"=T6."maximized", "display alerts? (F)"=TRUE, "report type"=Report_Type."Excel") -> ("report out"=w560:refnum<class "NI_report.lvclass">, "error out"=w562:errorcluster)  [unwired: 11 in]
            n215 = call <vilib>:"Excel Easy Title.vi"("report in"=w560, "title"=w558, "start (0, 0)"=cluster{"row":i32, "column":i32} {"row"=0, "column"=2}, "font"=T4 {"font name"="Times New Roman", "font size"=24.0, "bold"=1, "italic"=0, "underline"=0, "strike through"=0, "font color"=16777216}, "error in (no error)"=w562) -> ("report out"=w559:refnum<class "NI_report.lvclass">, "error out"=w561:errorcluster)  [unwired: 8 in, 1 out]
            n216 = property on="Log Table" class="Tbl (strict)"() -> ("Value"=w563:string[][])  [unwired: 2 in, 2 out]
            n217 = call-poly <vilib>:"Excel Easy Table.vi"("report in"=w559, "font"=T4 {"font name"="Times New Roman", "font size"=12.0, "bold"=0, "italic"=0, "underline"=0, "strike through"=0, "font color"=16777216}, "auto format (none)"=w547, "start (0, 0)"=cluster{"row":i32, "column":i32} {"row"=2, "column"=2}, "text data"=w563, "error in (no error)"=w561, "column headers"=string[] ["Log Catalog", "Date", "Time", "Description"]) -> ("error out"=w544:errorcluster)  [unwired: 4 in, 4 out]
          }
        }
        n218 = shared-variable ".\\Maintenance.lvlib\\error_64"(w297) -> ()  [unwired: 1 in, 1 out]
      }
      event "Search 1", "Search 2": Mouse Down {
        n219 = event-data() -> ()  [unwired: 1 in, 8 out]
        n220 = flat-sequence {
          tunnel: [w567] -> w564
          tunnel: w564 -> [w588]
          frame #0 {
            n221 = call "grading table searching.vi"() -> ()  [unwired: 12 in]
          }
          frame #1 {
            n222 = case shown="\"Grading Table\", Default" "Tab Control 1" {
              tunnel: [w572 w580] -> w568
              frame "Grading Table", Default {
                n223 = case shown="\"Disc 05\"" "Tab Control 2" {
                  tunnel: ["grading_disc_01" ("Connection Name") "grading_disc_02" ("Connection Name") "grading_disc_03" ("Connection Name") "grading_disc_04" ("Connection Name") "grading_disc_05" ("Connection Name") "grading_disc_06" ("Connection Name")] -> w572
                  frame "Disc 01", Default {
                  }
                  frame "Disc 02" {
                  }
                  frame "Disc 03" {
                  }
                  frame "Disc 04" {
                  }
                  frame "Disc 05" {
                  }
                  frame "Disc 06" {
                  }
                }
              }
              frame "Main Grading Table" {
                n224 = case shown="\"Disc 06\"" "Tab Control 3" {
                  tunnel: ["main_grading_group_disc_01" ("Connection Name") "main_grading_group_disc_02" ("Connection Name") "main_grading_group_disc_03" ("Connection Name") "main_grading_group_disc_04" ("Connection Name") "main_grading_group_disc_05" ("Connection Name") "main_grading_group_disc_06" ("Connection Name")] -> w580
                  frame "Disc 01", Default {
                  }
                  frame "Disc 02" {
                  }
                  frame "Disc 03" {
                  }
                  frame "Disc 04" {
                  }
                  frame "Disc 05" {
                  }
                  frame "Disc 06" {
                  }
                }
              }
            }
            n225 = shared-variable ".\\database.lvlib\\Query String"() -> (w571:string, error out=w566:errorcluster)  [unwired: 1 in]
            n226 = call "Query.vi"("Condition"=w571, "Error in"=w566, "Table Name"=w568, "Connection Name"="dsgs") -> ("Error out"=w565:errorcluster, "data"=w567:string[][])
            n227 = shared-variable ".\\Maintenance.lvlib\\error_65"(w565) -> ()  [unwired: 1 in, 1 out]
          }
          frame #2 {
            n228 = property on="Tab Control 1" class="TabCtl (strict)"() -> ("Value"=w589:T1)  [unwired: 2 in, 2 out]
            n229 = case shown="\"Main Grading Table\"" w589 {
              tunnel: w588 -> [w590 w610]
              frame "Grading Table", Default {
                n230 = property on="Tab Control 2" class="TabCtl (strict)"() -> ("Value"=w591:T2)  [unwired: 2 in, 2 out]
                n231 = case shown="\"Disc 01\", Default" w591 {
                  tunnel: w590 -> [w594 w596 w599 w602 w605 w608]
                  frame "Disc 01", Default {
                    n232 = Array Subset(array=w594, index (col)=1 ("index")) -> (→"Grading Table Disc 1":string[][])  [unwired: 3 in]
                  }
                  frame "Disc 02" {
                    n233 = Array Subset(array=w596, index (col)=1 ("index")) -> (→"Grading Table Disc 2":string[][])  [unwired: 3 in]
                  }
                  frame "Disc 03" {
                    n234 = Array Subset(array=w599, index (col)=1 ("index")) -> (→"Grading Table Disc 3":string[][])  [unwired: 3 in]
                  }
                  frame "Disc 04" {
                    n235 = Array Subset(array=w602, index (col)=1 ("index")) -> (→"Grading Table Disc 4":string[][])  [unwired: 3 in]
                  }
                  frame "Disc 05" {
                    n236 = Array Subset(array=w605, index (col)=1 ("index")) -> (→"Grading Table Disc 5":string[][])  [unwired: 3 in]
                  }
                  frame "Disc 06" {
                    n237 = Array Subset(array=w608, index (col)=1 ("index")) -> (→"Grading Table Disc 6":string[][])  [unwired: 3 in]
                  }
                }
              }
              frame "Main Grading Table" {
                n238 = property on="Tab Control 3" class="TabCtl (strict)"() -> ("Value"=w611:T2)  [unwired: 2 in, 2 out]
                n239 = case shown="\"Disc 06\"" w611 {
                  tunnel: w610 -> [w613 w616 w619 w622 w625 w628]
                  frame "Disc 01", Default {
                    n240 = Array Subset(array=w613, index (col)=1 ("index")) -> (→"Main Grading Table Disc 1":string[][])  [unwired: 3 in]
                  }
                  frame "Disc 02" {
                    n241 = Array Subset(array=w616, index (col)=1 ("index")) -> (→"Main Grading Table Disc 2":string[][])  [unwired: 3 in]
                  }
                  frame "Disc 03" {
                    n242 = Array Subset(array=w619, index (col)=1 ("index")) -> (→"Main Grading Table Disc 3":string[][])  [unwired: 3 in]
                  }
                  frame "Disc 04" {
                    n243 = Array Subset(array=w622, index (col)=1 ("index")) -> (→"Main Grading Table Disc 4":string[][])  [unwired: 3 in]
                  }
                  frame "Disc 05" {
                    n244 = Array Subset(array=w625, index (col)=1 ("index")) -> (→"Main Grading Table Disc 5":string[][])  [unwired: 3 in]
                  }
                  frame "Disc 06" {
                    n245 = Array Subset(array=w628, index (col)=1 ("index")) -> (→"Main Grading Table Disc 6":string[][])  [unwired: 3 in]
                  }
                }
              }
            }
          }
        }
      }
      event "Grading Table Disc 1": Mouse Down {
        n246 = event-data() -> ("CtlRef"=w637:refnum<vi>)  [unwired: 1 in, 7 out]
        n247 = property on="Property Node" class="Tbl (strict)"(reference=w637) -> ("Value"=w636:string[][], "Selection Start"=w639:T7)  [unwired: 1 in, 2 out]
        n248 = Unbundle By Name(w639) -> ("Row"=w634:i32)
        n249 = Matrix Size(0:w636) -> (1:w635:i32)  [unwired: 1 out]
        n250 = Greater Or Equal?(x=w635, y=w634) -> (x >= y?=w633:bool)
        n251 = Select(t=T7 {"Row"=1, "Column"=14} ("Selection Size"), s=w633, f=T7 {"Row"=0, "Column"=0}) -> (s? t:f=w631:T7)
        n252 = Bundle("Row"=w634, "Row"=0) -> (w641:cluster{"Row":i32, "Row":i32})  [unwired: 1 in]
        n253 = property on="Property Node" class="Tbl (strict)"(reference=w637, "Selection Color"=u32 16711680, "Selection Size"=w631, "Selection Start"=w641) -> ()  [unwired: 1 in, 2 out]
      }
      event "Main Grading Table Disc 1", "Main Grading Table Disc 2", "Main Grading Table Disc 3", "Main Grading Table Disc 4", "Main Grading Table Disc 5": Mouse Down {
        n254 = event-data() -> ("CtlRef"=w649:refnum<vi>)  [unwired: 1 in, 7 out]
        n255 = property on="Property Node" class="Tbl (strict)"(reference=w649) -> ("Value"=w644:string[][], "Selection Start"=w651:T7)  [unwired: 1 in, 2 out]
        n256 = Unbundle By Name(w651) -> ("Row"=w642:i32)
        n257 = Matrix Size(0:w644) -> (1:w648:i32)  [unwired: 1 out]
        n258 = Greater Or Equal?(x=w648, y=w642) -> (x >= y?=w647:bool)
        n259 = Bundle("Row"=w642, "Row"=0) -> (w653:cluster{"Row":i32, "Row":i32})  [unwired: 1 in]
        n260 = Select(t=T7 {"Row"=1, "Column"=8} ("Selection Size"), s=w647, f=T7 {"Row"=0, "Column"=0}) -> (s? t:f=w643:T7)
        n261 = property on="Property Node" class="Tbl (strict)"(reference=w649, "Selection Color"=u32 16711680, "Selection Size"=w643, "Selection Start"=w653) -> ()  [unwired: 1 in, 2 out]
      }
      event "Log Catalog Table", "Log Table", "User Table": Mouse Down {
        n262 = event-data() -> ("CtlRef"=w661:refnum<vi>)  [unwired: 1 in, 7 out]
        n263 = property on="Property Node" class="Tbl (strict)"(reference=w661) -> ("Value"=w656:string[][], "Selection Start"=w663:T7)  [unwired: 1 in, 2 out]
        n264 = Unbundle By Name(w663) -> ("Row"=w655:i32)
        n265 = Matrix Size(0:w656) -> (1:w660:i32)  [unwired: 1 out]
        n266 = Greater Or Equal?(x=w660, y=w655) -> (x >= y?=w659:bool)
        n267 = Bundle("Row"=w655, "Row"=0) -> (w665:cluster{"Row":i32, "Row":i32})  [unwired: 1 in]
        n268 = Select(t=T7 {"Row"=1, "Column"=4} ("Selection Size"), s=w659, f=T7 {"Row"=0, "Column"=0}) -> (s? t:f=w654:T7)
        n269 = property on="Property Node" class="Tbl (strict)"(reference=w661, "Selection Color"=u32 16711680, "Selection Size"=w654, "Selection Start"=w665) -> ()  [unwired: 1 in, 2 out]
      }
      event "Search 3": Mouse Down {
        n270 = event-data() -> ()  [unwired: 1 in, 8 out]
        n271 = flat-sequence {
          frame #0 {
            n272 = call "log table searching.vi"() -> ()  [unwired: 12 in]
          }
          frame #1 {
            n273 = shared-variable ".\\database.lvlib\\Query String"() -> (w672:string, error out=w667:errorcluster)  [unwired: 1 in]
            n274 = call "Query.vi"("Condition"=w672, "Error in"=w667, "Table Name"="log_table", "Connection Name"="dsgs") -> ("Error out"=w666:errorcluster, "data"=w670:string[][])
            n275 = shared-variable ".\\Maintenance.lvlib\\error_66"(w666) -> ()  [unwired: 1 in, 1 out]
            n276 = Array Subset(array=w670, index (col)=1 ("index")) -> (→"Log Table":string[][])  [unwired: 3 in]
          }
        }
      }
      event "Tab Control 1": Mouse Down {
        n277 = event-data() -> ("CtlRef"=w675:refnum<vi>)  [unwired: 1 in, 7 out]
        n278 = property class="TabCtl (strict)"(reference=w675) -> ("Value"=w674:T1)  [unwired: 1 in, 2 out]
        n279 = case shown="\"User Table\", Default" w674 {
          frame "Log Table" {
            n280 = call "Query.vi"("Table Name"="log_catalog", "Connection Name"="dsgs") -> ("Error out"=w676:errorcluster, "data"=→"Log Catalog Table":string[][])  [unwired: 2 in]
            n281 = shared-variable ".\\Maintenance.lvlib\\error_67"(w676) -> ()  [unwired: 1 in, 1 out]
          }
          frame "User Table", Default {
            n282 = call "Query.vi"("Table Name"="user_table", "Connection Name"="dsgs") -> ("Error out"=w680:errorcluster, "data"=w688:string[][])  [unwired: 2 in]
            n283 = Index Array(array=w688, index (col) #1=0 ("disabled index (col)"), index (col) #3=3 ("index (col)")) -> (element #1=w685:string[], element #2=w684:string[], element #3=w683:string[])  [unwired: 4 in]
            n284 = shared-variable ".\\Maintenance.lvlib\\error_68"(w680) -> ()  [unwired: 1 in, 1 out]
            n285 = Build Array(w685, w684, w683) -> (w682:string[][])
            n286 = Transpose 2D Array(2D array=w682) -> (transposed array=→"User Table":string[][])
          }
        }
      }
      event Timeout {
        n287 = event-data() -> ()  [unwired: 1 in, 3 out]
        n288 = control-ref of="This VI"() -> (w691:refnum<vi>)
        n289 = shared-variable ".\\database.lvlib\\ReportThisVI"(w691) -> ()  [unwired: 1 in, 1 out]
      }
    }
  }
  n290 = property on="Main Grading Table Disc 1" class="Tbl (strict)"("BuiltInMouseWheelSupport"=w1) -> ()  [unwired: 2 in, 2 out]
  n291 = property on="Main Grading Table Disc 2" class="Tbl (strict)"("BuiltInMouseWheelSupport"=w1) -> ()  [unwired: 2 in, 2 out]
  n292 = property on="Main Grading Table Disc 3" class="Tbl (strict)"("BuiltInMouseWheelSupport"=w1) -> ()  [unwired: 2 in, 2 out]
  n293 = property on="Main Grading Table Disc 4" class="Tbl (strict)"("BuiltInMouseWheelSupport"=w1) -> ()  [unwired: 2 in, 2 out]
  n294 = property on="Main Grading Table Disc 5" class="Tbl (strict)"("BuiltInMouseWheelSupport"=w1) -> ()  [unwired: 2 in, 2 out]
  n295 = property on="User Table" class="Tbl (strict)"("BuiltInMouseWheelSupport"=w1) -> ()  [unwired: 2 in, 2 out]
  n296 = property on="Log Table" class="Tbl (strict)"("BuiltInMouseWheelSupport"=w1) -> ()  [unwired: 2 in, 2 out]
  n297 = property on="Log Catalog Table" class="Tbl (strict)"("BuiltInMouseWheelSupport"=w1) -> ()  [unwired: 2 in, 2 out]
  n298 = property on="Grading Table Disc 1" class="Tbl (strict)"("BuiltInMouseWheelSupport"=w1) -> ()  [unwired: 2 in, 2 out]
  n299 = property on="Grading Table Disc 2" class="Tbl (strict)"("BuiltInMouseWheelSupport"=w1) -> ()  [unwired: 2 in, 2 out]
  n300 = property on="Grading Table Disc 3" class="Tbl (strict)"("BuiltInMouseWheelSupport"=w1) -> ()  [unwired: 2 in, 2 out]
  n301 = property on="Grading Table Disc 4" class="Tbl (strict)"("BuiltInMouseWheelSupport"=w1) -> ()  [unwired: 2 in, 2 out]
  n302 = property on="Grading Table Disc 5" class="Tbl (strict)"("BuiltInMouseWheelSupport"=w1) -> ()  [unwired: 2 in, 2 out]
  n303 = property on="Grading Table Disc 6" class="Tbl (strict)"("BuiltInMouseWheelSupport"=w1) -> ()  [unwired: 2 in, 2 out]
